vi "DB UI - Config.vi"() -> ()   [LabVIEW 2013]
uses:
  <vilib>/event_ctls.llb/lveventtype.ctl
  Controls/Combo Box.ctl
  <vilib>/Utility/miscctls.llb/LVRowAndColumnTypeDef.ctl
  <vilib>/Utility/miscctls.llb/LVRowAndColumnUnsignedTypeDef.ctl
  Controls/DB - Table Group Enum.ctl
  <vilib>/Utility/miscctls.llb/LVPointTypeDef.ctl
  Controls/DB - OpenClose.ctl
  Controls/DB - Config Table Enum.ctl
  Controls/MCListbox - Enum.ctl
  Controls/Global SRTRS.vi
  Controls/Global CMS.vi
  Controls/Global AMS.vi
  <vilib>/addons/database/Connection.llb/DB Tools Open Connec (String).vi
  <vilib>/addons/database/Connection.llb/Conn Execute.vi
  <vilib>/addons/database/Recordset.llb/Rec Fetch Recordset Data (R).vi
  <vilib>/addons/database/Recordset.llb/Rec Destroy - Connection.vi
  <vilib>/addons/database/_DB Variant To Data/Database Variant To Data.xnode
  <vilib>/addons/database/NI_Database_API.lvlib
panel:
  in  "Application":string
  in  "Records [CaptionOnly]":string caption="Records"
  in  "Header [CaptionOnly]":string caption="Header"
  in  "Tab Control":enum32{"Debug"}(tab)
  out "MHandler":errorcluster
  out "Connection Information":T1={"Connection "="SQL Server 32bit HPEnvy", "Username"="admin", "Password"="admin123"}
  in  "Stop Button":bool
  in  "# of Columns":i32=5
  out "Primary Keys":string[](array[string])=["OrderNo"]
  out "Foreign Keys":string[](array[string])=["OrderNo"]
  out "1st Primary KEY":string
  out "datetime string":string
  out "Changed":bool
  out "SQL Query":string
  out "Extra Event From \"Select Foreign Key\"":bool
  out "IDENTITY COLUMN":string
  out "New Record in UI not in DB":bool
  out "DB.Config.TableGroupType":string="SRTRS.Config.TableGroupType"
  out "Active Cell:Active Cell":T2
  out "# of Columns in DB Table":i32
  out "DB.Config.TableGroup":string="SRTRS.Config.TableGroup"
  in  "CellBG New Cells":u32(colorbox)=16777225
  in  "CellBG Unused Cells":u32(colorbox)=16777238
  in  "CellBG ColHdrs":u32(colorbox)=11776947
  out "Statemachine":errorcluster
  out "Close":errorcluster
  out "Property Node":errorcluster
  out "Foreign Key Selected":string
  out "Type":T3=enum."Value Change"
  out "MCListBox EditCell, Extra Event From  \"Select Foreign Key\"":u32
  out "DB":errorcluster
  in  "Copy":bool
  in  "Database Group":string(combo)
  in  "Save":bool caption="Setup Save"
  in  "Delete":bool caption="Setup Save"
  in  "New":bool caption="Setup Save"
  out "Table Description":string
  in  "Table Name":T4
  in  "Include Inactive":bool
  in  "First Button":bool
  in  "Last Button":bool
  in  "Select Foreign Key":string(combo)="bee"
  in  "Current Record":i32
  in  "Previous Button":bool
  in  "Next Button":bool
  out "Record Count":i32
  in  "Multicolumn Listbox":i32(listbox)=3
  # "Cannot be placed in Tabs, because calling VI only looking at first level."
  # "/"
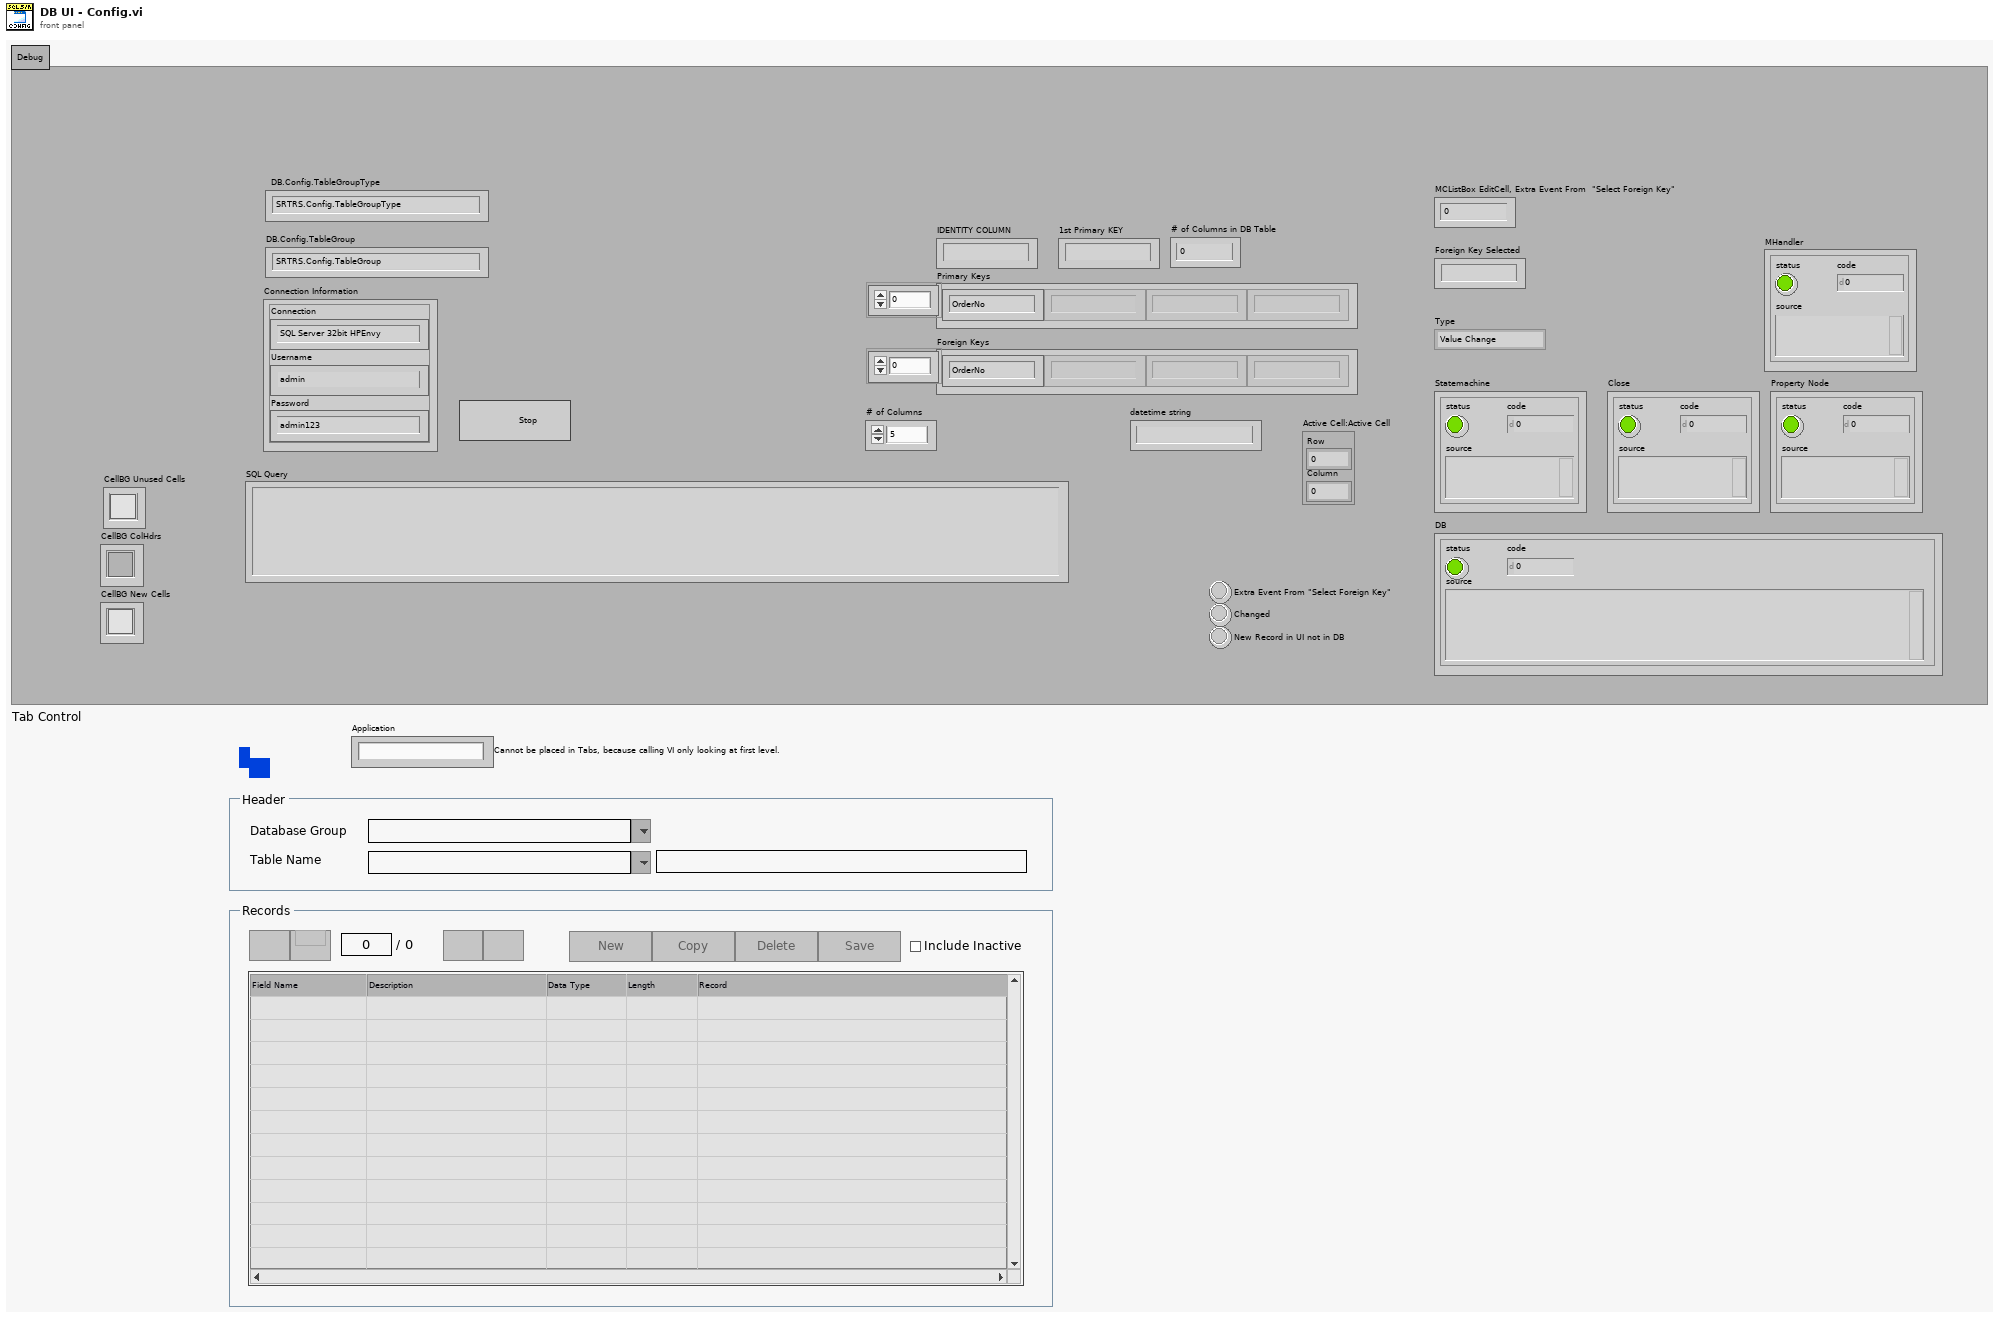
[diagram p1: front panel]
types:
  T1 = cluster{"Connection ":string, "Username":string, "Password":string}
  T2 = typedef "LVRowAndColumnTypeDef.ctl" = cluster{"Row":i32, "Column":i32}
  T3 = typedef "lveventtype.ctl" = enum32{"Null", "Timeout", "Annotation Menu Selection", "Annotation Menu Selection?", "App Instance Close", "App Instance Close?", "Autoscale Range Change", "Bookmark Info Change", "Cell Edit", "Cell Edit?", "Cursor Grab", "Cursor Grab?", "Cursor Menu Selection", "Cursor Menu Selection?", "Cursor Move", "Cursor Release", "Data Change", "Direction Change", "Display State Change", "Drag Ended", "Drag Enter", "Drag Leave", "Drag Over", "Drag Source Update", "Drag Starting", "Drag Starting?", "Drop", "Exec State Change", "Key Down", "Key Down?", "Key Repeat", "Key Repeat?", "Key Up", "Listbox Double Click", "Menu Activation?", "Menu Selection (App)", "Menu Selection? (App)", "Menu Selection (User)", "Mouse Down", "Mouse Down?", "Mouse Enter", "Mouse Leave", "Mouse Move", "Mouse Up", "Mouse Wheel", "NI Security User Change (App)", "Pane Size", "Panel Close", "Panel Close?", "Panel Resize", "Plot Attribute Change", "Scale Range Change", "Shortcut Menu Activation?", "Shortcut Menu Selection (App)", "Shortcut Menu Selection? (App)", "Shortcut Menu Selection (User)", "Tree Double Click", "Tree Drag", "Tree Drag?", "Tree Drop", "Tree Drop?", "Tree Item Close", "Tree Item Close?", "Tree Item Open", "Tree Item Open?", "User Event", "Value Change"}
  T4 = typedef "Combo Box.ctl" = string
  T5 = typedef "DB - OpenClose.ctl" = cluster{"Open":bool, "Close":bool}
  T6 = typedef "LVPointTypeDef.ctl" = cluster{"Horizontal":i16, "Vertical":i16}
  T7 = typedef "DB - Table Group Enum.ctl" = enum16{"SELECT [Description]", "SELECT [TableGroupId]"}
  T8 = typedef "LVRowAndColumnUnsignedTypeDef.ctl" = cluster{"Row":u32, "Column":u32}
  T9 = enum8{"Enabled", "Disabled", "Disabled and Grayed Out"}
  T10 = typedef "Connection Information Cluster.ctl" = cluster{"Connection ":string, "Username":string, "Password":string}
  T11 = typedef "NI_Database_API.lvlib/Conn ObjectReference.ctl" = refnum<k1>
  T12 = typedef "DB - Config Table Enum.ctl" = enum16{"Column Name", "Description", "Type", "Length", "Value (Data)"}
  T13 = typedef "MCListbox - Enum.ctl" = enum16{"Initial (KD?)", "Initial Text", "B4 <Return>", "Now", "Max row count", "Mandatory Fields", "Data Type", "Stored Row, Col, Color"}
  T14 = enum16{"Find FK's Primary Schema.Table", "Find PK's Foreign Schema.Table"}
  T15 = typedef "eventvkey.ctl" = enum16{"ASCII", "Enter", "Return", "Shift", "Ctrl", "Alt", "Cmd", "Opt", "Caps", "NumLock", "Clear", "Break", "Up", "Down", "Left", "Right", "Insert", "Delete", "Home", "End", "PageUp", "PageDown", "Escape", "Help", "Pause", "ScrollLock", "F1", "F2", "F3", "F4", "F5", "F6", "F7", "F8", "F9", "F10", "F11", "F12", "F13", "F14", "F15", "F16", "F17", "F18", "F19", "F20", "F21", "F22", "F23", "F24", "Play", "VolumeUp", "VolumeDown", "Mute", "Two Byte Char"}
  T16 = typedef "LVPoint32TypeDef.ctl" = cluster{"Horizontal":i32, "Vertical":i32}
  T17 = typedef "NI_Database_API.lvlib/Rec ObjectReference.ctl" = refnum<k1>
  T18 = typedef "DB - DB.Schema.Table.ctl" = cluster{"DB":string, "Schema":string, "Table":string}
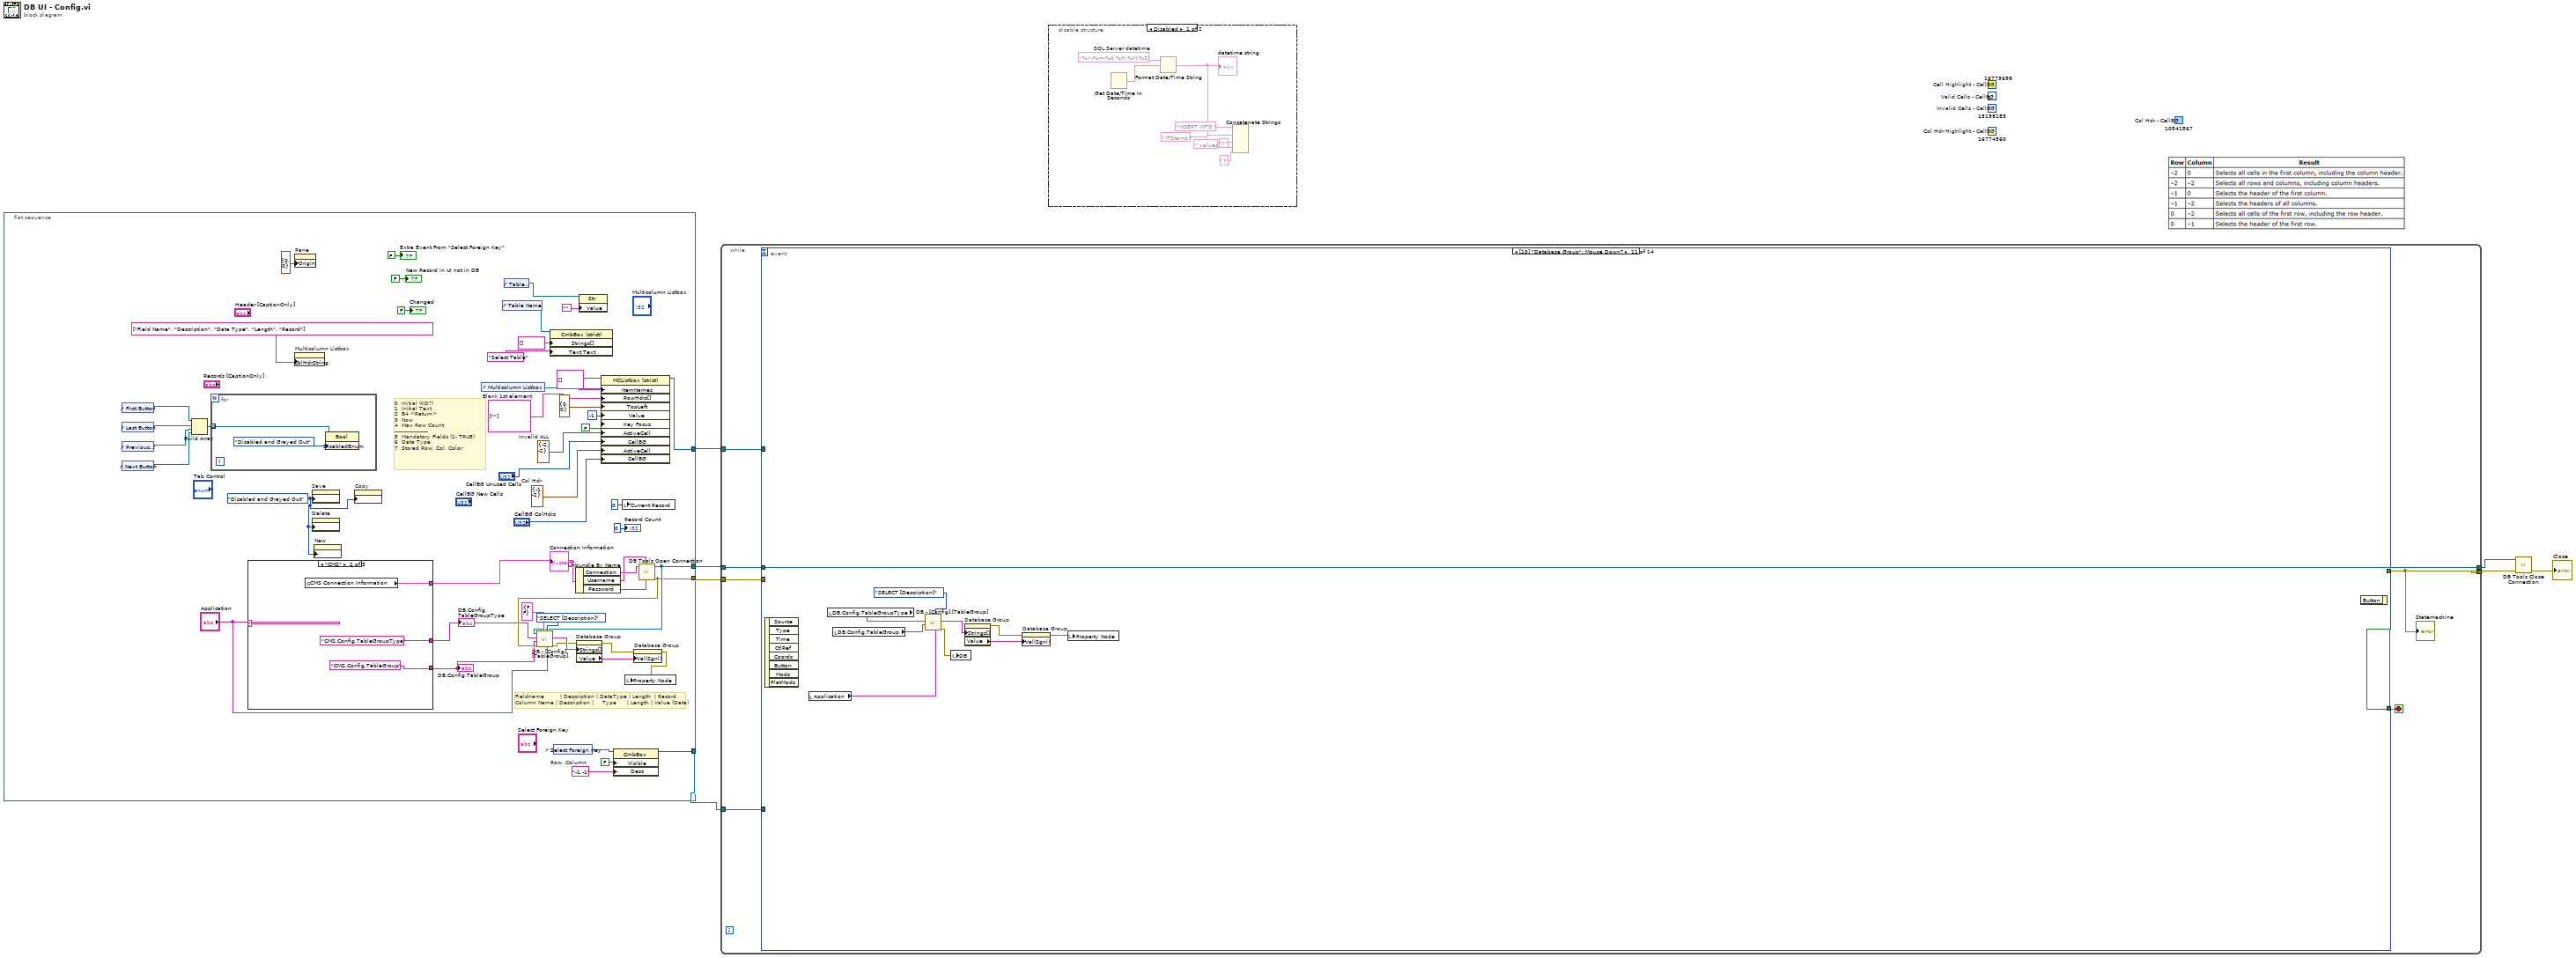
[diagram p0: block diagram]
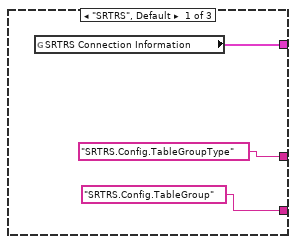
[diagram p3: hidden frame]
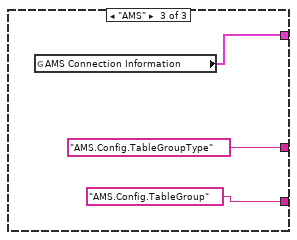
[diagram p4: hidden frame]
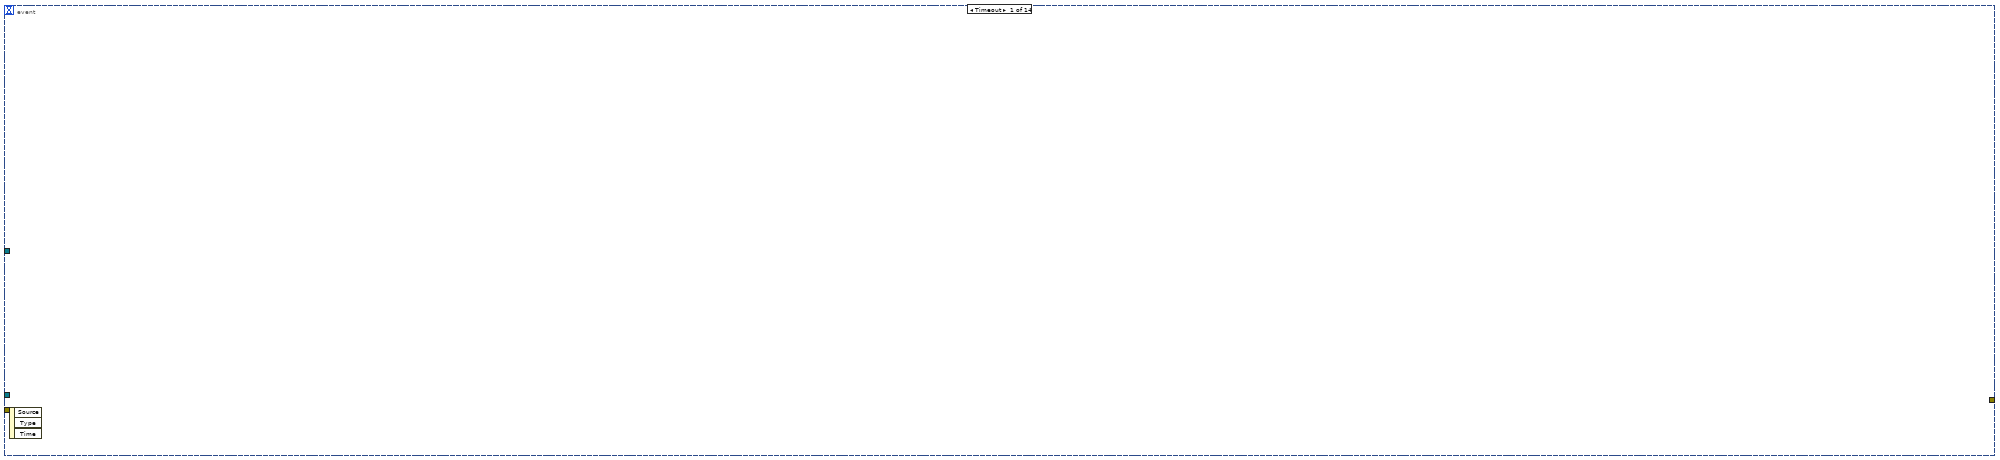
[diagram p5: hidden frame]
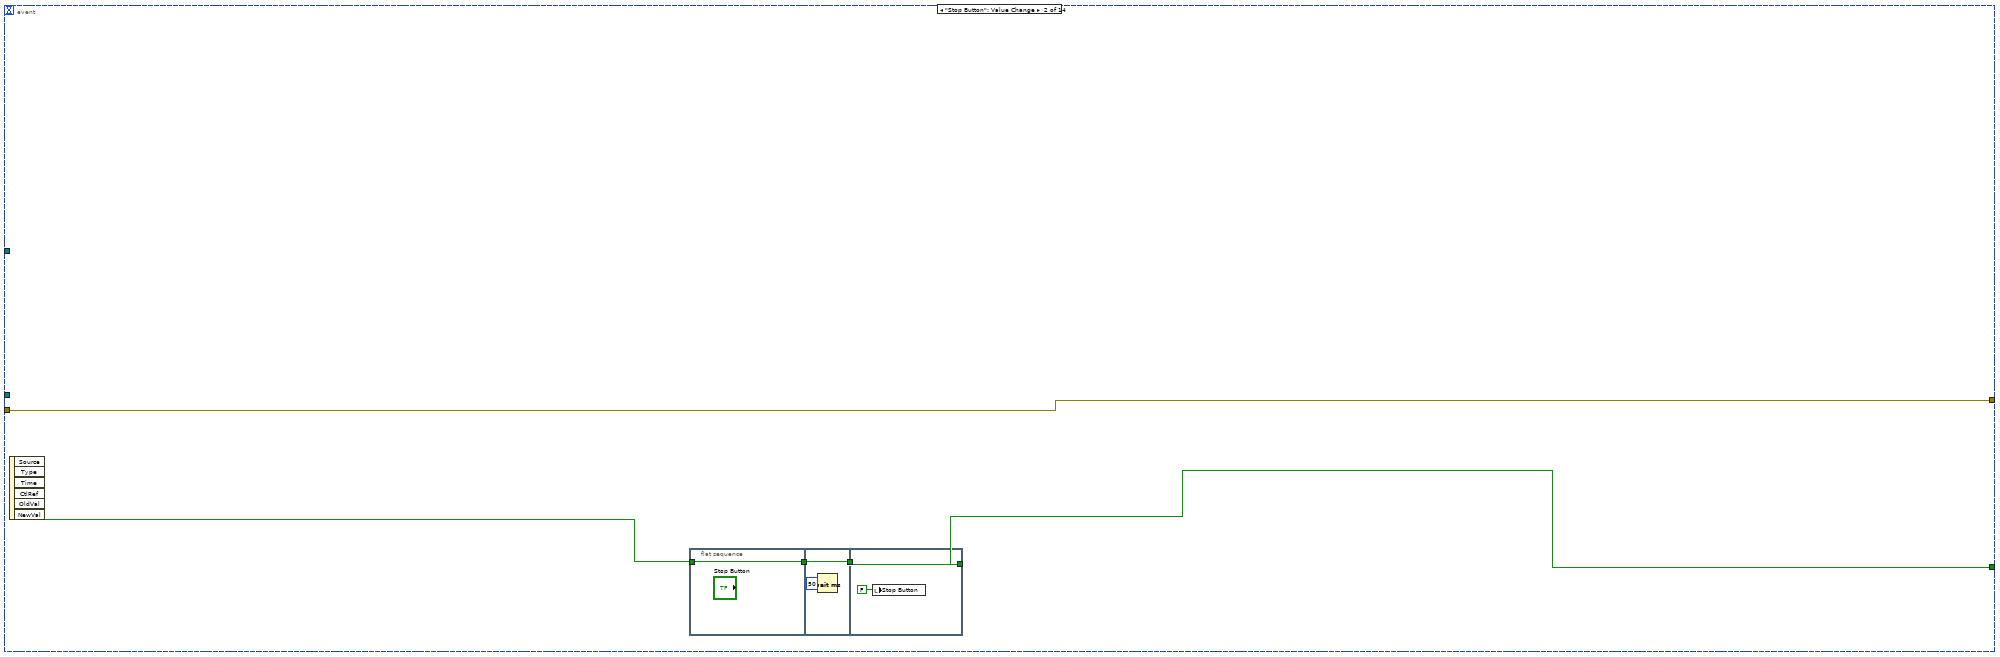
[diagram p6: hidden frame]
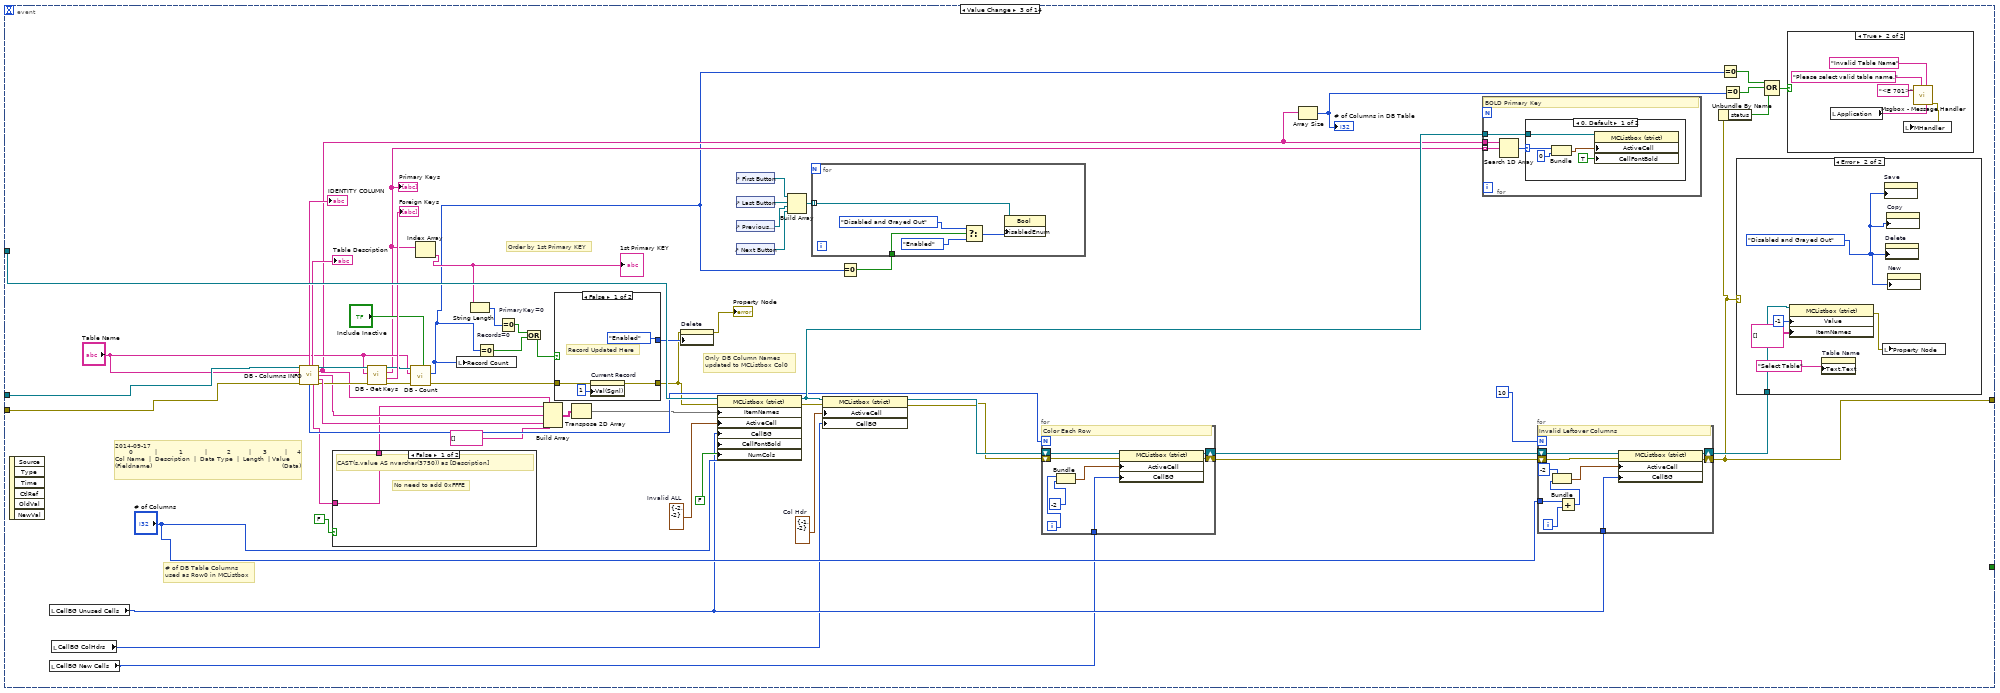
[diagram p7: hidden frame]
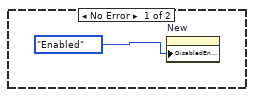
[diagram p9: hidden frame]
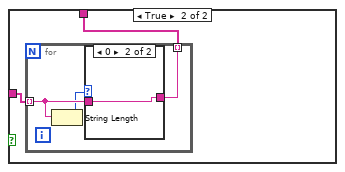
[diagram p10: hidden frame]
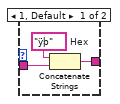
[diagram p11: hidden frame]
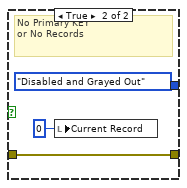
[diagram p12: hidden frame]
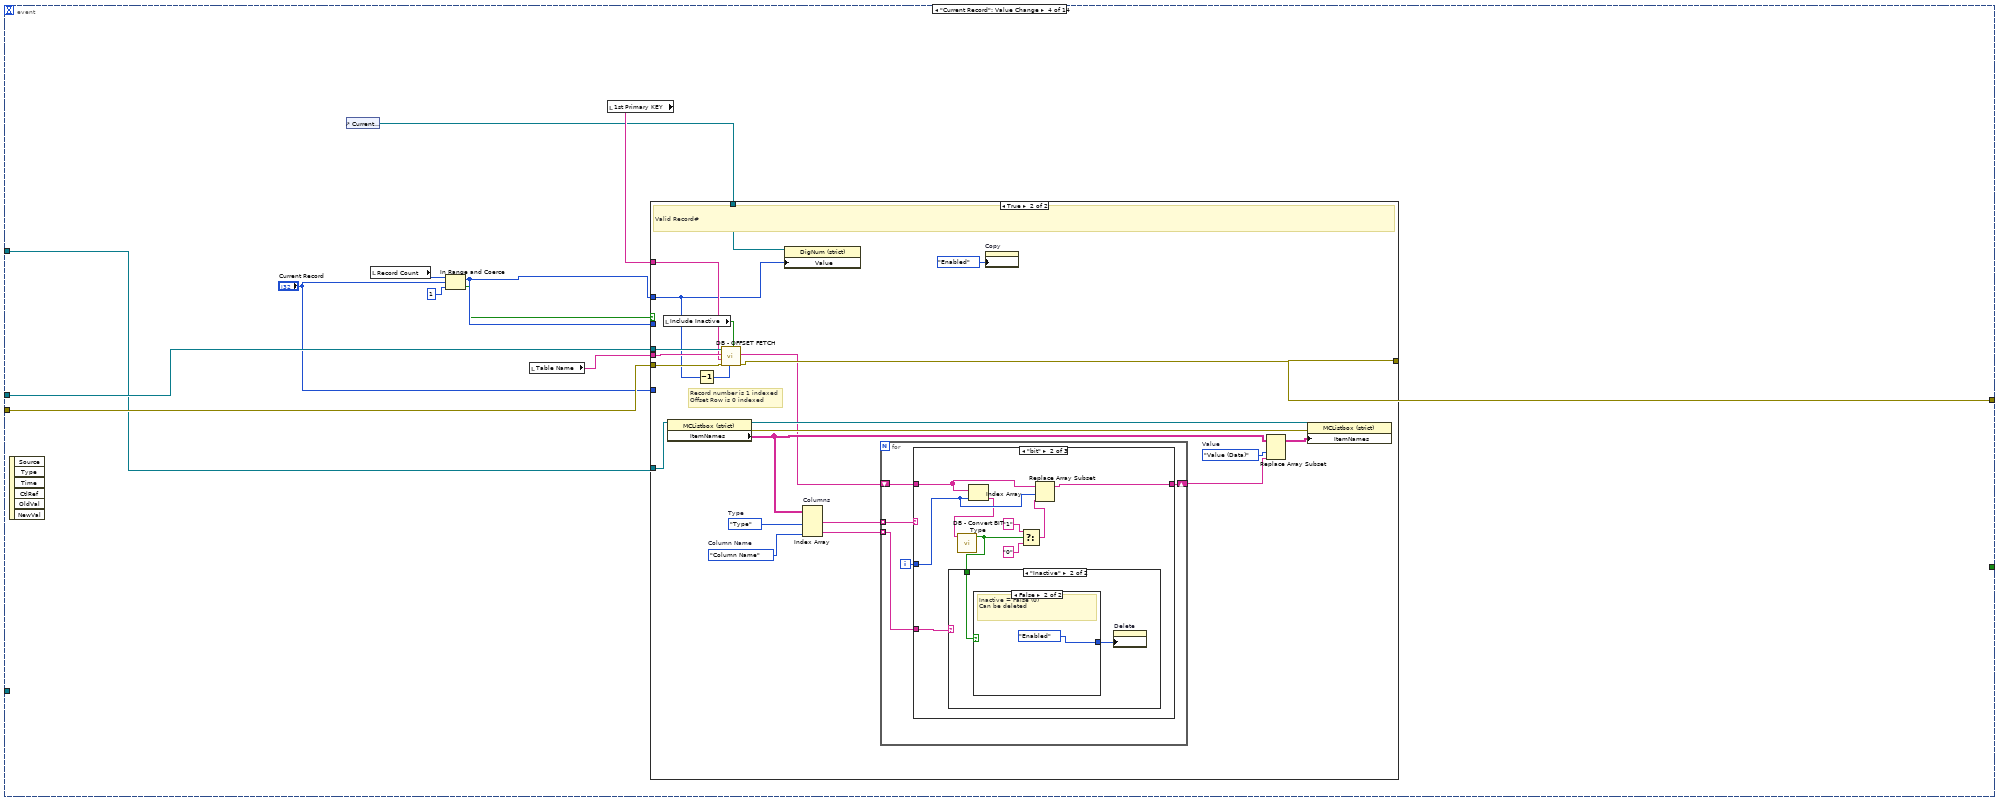
[diagram p14: hidden frame]
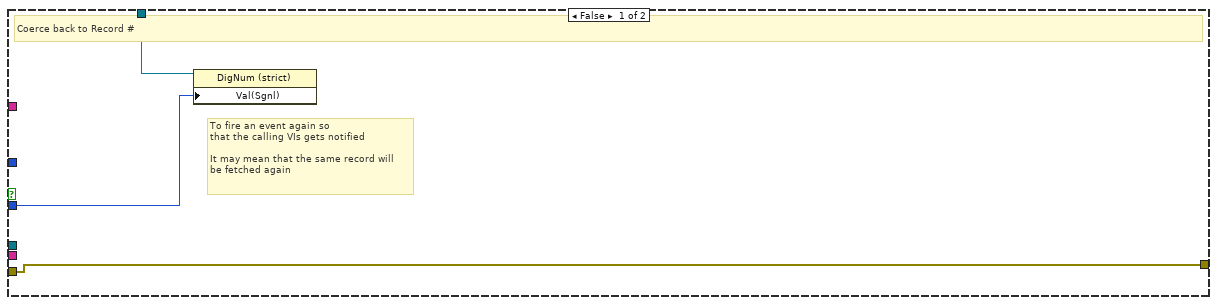
[diagram p15: hidden frame]
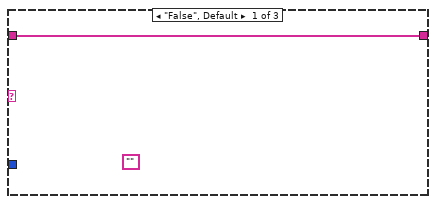
[diagram p16: hidden frame]
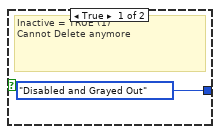
[diagram p18: hidden frame]
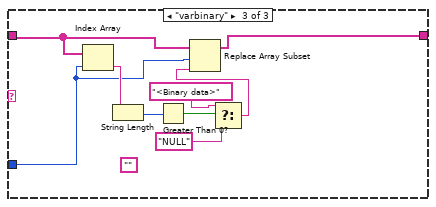
[diagram p19: hidden frame]
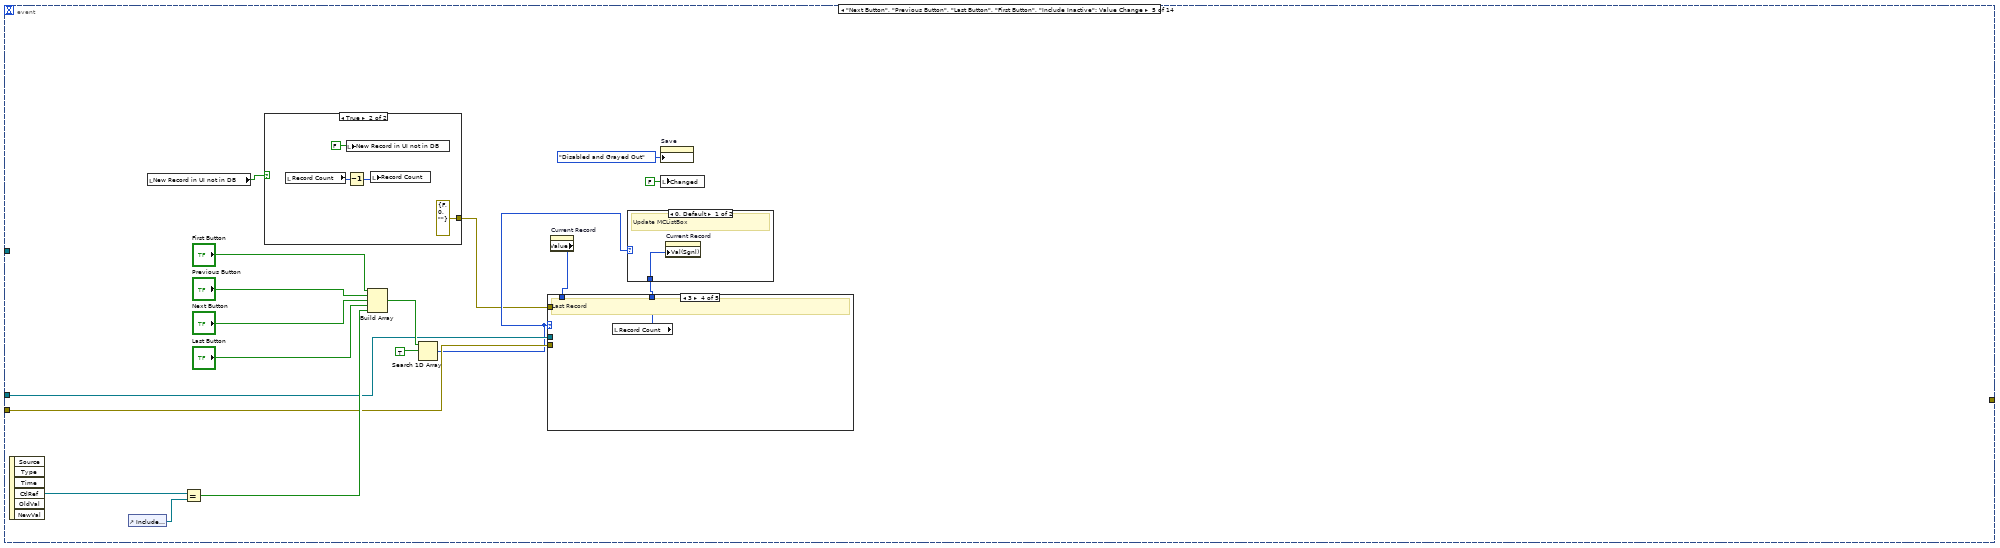
[diagram p20: hidden frame]
diagram:
  (unwired) u32 10541567  # Col Hdr - CellBG
  (unwired) u32 16777226  # Valid Cells - CellBG
  (unwired) u32 15198183  # Invalid Cells - CellBG
  (unwired) u32 16774560  # Col Hdr Highlight - CellBG
  (unwired) u32 16773698  # Cell Highlight - CellBG
  n1 = flat-sequence {
    tunnel: [w18] -> w7
    tunnel: [w52] -> w4
    tunnel: [w17] -> w3
    tunnel: [w49] -> w2
    frame #0 {
      w26 = T2 {"Row"=-1, "Column"=-2}  # Col Hdr
      w27 = T2 {"Row"=-2, "Column"=-2}  # Invalid ALL
      w28 = string[] [""]  # Blank 1st element
      w9 = T9."Disabled and Grayed Out" ("Disabled")
      w47 = "-1,-1"  # Row, Column
      # "Fieldname         | Description | DataType | Length  | Record \nColumn Name | Description |     Type      | Length | Value (Data)"
      # "0  Initial (KD?)\n1  Initial Text\n2  B4 <Return>\n3  Now\n4  Max Row Count\n-------------------\n5  Mandatory Fields (1- TRUE)\n6  Data Type\n7  Stored Row, Col, Color"
      n2 = control-ref of="First Button"() -> (w43:refnum<vi>)
      n3 = control-ref of="Last Button"() -> (w42:refnum<vi>)
      n4 = control-ref of="Previous Button"() -> (w41:refnum<vi>)
      n5 = control-ref of="Next Button"() -> (w40:refnum<vi>)
      n6 = Build Array(w43, w42, w41, w40) -> (w44:refnum<vi>[])
      n7 = for {
        tunnel: w44 -> [w67] mode=indexing
        n8 = property class="Bool"(reference=w67, "DisabledEnum"=T9."Disabled and Grayed Out" ("Disabled")) -> ()  [unwired: 1 in, 2 out]
      }
      n9 = case shown="\"CMS\"" "Application" {
        tunnel: [w59 w62 w63] -> w21
        tunnel: ["SRTRS.Config.TableGroupType" ("DB.Schema.Table\nDB.Config.TableGroupType") "CMS.Config.TableGroupType" ("DB.Schema.Table\nDB.Config.TableGroupType") "AMS.Config.TableGroupType" ("DB.Schema.Table\nDB.Config.TableGroupType")] -> w20
        tunnel: ["SRTRS.Config.TableGroup" ("DB.Schema.Table\nDB.Config.TableGroup") "CMS.Config.TableGroup" ("DB.Schema.Table\nDB.Config.TableGroup") "AMS.Config.TableGroup" ("DB.Schema.Table\nDB.Config.TableGroup")] -> w10
        frame "SRTRS", Default {
          n10 = global read "Global SRTRS.vi" "SRTRS Connection Information"() -> (w59:T10)
        }
        frame "CMS" {
          n11 = global read "Global CMS.vi" "CMS Connection Information"() -> (w62:T10)
        }
        frame "AMS" {
          n12 = global read "Global AMS.vi" "AMS Connection Information"() -> (w63:T10)
        }
      }
      "Connection Information" <- w21
      "DB.Config.TableGroupType" <- w20
      "DB.Config.TableGroup" <- w10
      n13 = property on="Pane" class="Pane"("Origin"=T6 {"Horizontal"=0, "Vertical"=0}) -> ()  [unwired: 2 in, 2 out]
      n14 = property on="Multicolumn Listbox" class="MCListbox (strict)"("ColHdrString"=string[] ["Field Name", "Description", "Data Type", "Length", "Record"] ("Column Header Strings[]")) -> ()  [unwired: 2 in, 2 out]
      n15 = property on="Save" class="Bool"("DisabledEnum"=w9) -> ()  [unwired: 2 in, 2 out]
      n16 = property on="Delete" class="Bool"("DisabledEnum"=w9) -> ()  [unwired: 2 in, 2 out]
      n17 = property on="New" class="Bool"("DisabledEnum"=w9) -> ()  [unwired: 2 in, 2 out]
      n18 = property on="Copy" class="Bool"("DisabledEnum"=w9) -> ()  [unwired: 2 in, 2 out]
      n19 = control-ref of="Multicolumn Listbox"() -> (w22:refnum<vi>)
      n20 = control-ref of="Table Name"() -> (w39:refnum<vi>)
      n21 = control-ref of="Table Description"() -> (w37:refnum<vi>)
      n22 = property on="Property Node" class="CmbBox (strict)"(reference=w39, "Strings[]"=string[] [] ("Strings []"), "Text.Text"="Select Table") -> ()  [unwired: 1 in, 2 out]
      n23 = control-ref of="Select Foreign Key"() -> (w50:refnum<vi>)
      n24 = Unbundle By Name(w21) -> ("Connection"=w55:string, "Username"=w54:string, "Password"=w53:string)
      n25 = property on="Property Node" class="Str"(reference=w37, "Value"="") -> ()  [unwired: 1 in, 2 out]
      n26 = property on="Property Node" class="MCListbox (strict)"(reference=w22, "ItemNames"=string[][] [] ("Item Names"), "RowHdrs[]"=w28, "TopLeft"=T8 {"Row"=0, "Column"=0} ("Top Left Visible Cell"), "Value"=-1, "Key Focus"=FALSE, "ActiveCell"=w27, "CellBG"="CellBG Unused Cells", "ActiveCell"=w26, "CellBG"="CellBG ColHdrs") -> (reference out=w52:refnum<vi>)  [unwired: 1 in, 1 out]
      n27 = property class="CmbBox"(reference=w50, "Visible"=FALSE, "Desc"=w47) -> (reference out=w49:refnum<vi>)  [unwired: 1 in, 1 out]
      n28 = local write "Current Record"(0 ("Current Record")) -> ()
      n29 = call-poly <vilib>:"DB Tools Open Connection.vi"("password"=w53, "userID"=w54, "connection information"=w55) -> ("error out"=w17:errorcluster, "connection reference"=w18:T11)  [unwired: 5 in]
      n30 = call "DB - [Config].[TableGroup].vi"("Application"="Application", "Table Group Enum"=DB_-_Table_Group_Enum."SELECT [Description]", "DB Connection"=T5 {"Open"=FALSE, "Close"=FALSE}, "error in (no error)"=w17, "DB.Config.TableGroup"=w10, "DB.Config.TableGroupType"=w20, "connection reference"=w18) -> ("SUMMARY"=w16:errorcluster, "data"=w31:string[])  [unwired: 2 in, 1 out]
      n31 = property on="Database Group" class="CmbBox"(error in=w16, "Strings[]"=w31) -> (error out=w25:errorcluster, "Value"=w24:string)  [unwired: 1 in, 1 out]
      n32 = property on="Database Group" class="CmbBox"(error in=w25, "Val(Sgnl)"=w24) -> (error out=w15:errorcluster)  [unwired: 1 in, 1 out]
      n33 = local write "Property Node"(w15) -> ()
      "Extra Event From \"Select Foreign Key\"" <- FALSE ("Extra Event From \"Select Foreign Key Value Changed\"")
      "Record Count" <- 0 ("Record Count")
      "New Record in UI not in DB" <- FALSE ("New Record in UI not in DB")
      "Changed" <- FALSE ("Changed")
    }
  }
  n34 = while {
    tunnel: w7 -> [w69]
    tunnel: [w69] -> w6
    tunnel: [w68] -> w5
    tunnel: w3 -> [w72]
    tunnel: w4 -> [w71]
    tunnel: w2 -> [w70]
    stop <- w73 stop-if-true
    n35 = event shown="[10] \"Database Group\": Mouse Down?" {
      selector: _ -> [_ _ _ _ _ _ _ _ _ _ _ _ _ _]
      dyn-events: _ -> [_ _ _ _ _ _ _ _ _ _ _ _ _ _]
      timeout: _ -> [_ _ _ _ _ _ _ _ _ _ _ _ _ _]
      tunnel: [_ w76 _ _ _ _ _ _ _ _ _ _ _ _] -> w73
      tunnel: w69 -> [_ _ w129 w216 w275 _ w367 _ _ w619 _ _ _ w806]
      tunnel: [_ w78 w90 w213 _ _ _ _ _ w581 _ _ _ _] -> w68
      tunnel: w72 -> [_ w78 w126 w215 w274 _ w366 _ _ _ _ _ _ _]
      tunnel: w71 -> [_ _ w138 w212 _ w308 _ _ w535 _ _ w727 w779 _]
      tunnel: w70 -> [_ _ _ _ _ _ w376 _ _ _ _ _ w781 _]
      event Timeout {
        n36 = event-data() -> ()  [unwired: 1 in, 3 out]
      }
      event "Stop Button": Value Change {
        n37 = event-data() -> ("NewVal"=w77:bool)  [unwired: 1 in, 5 out]
        n38 = flat-sequence {
          tunnel: w77 -> [w79]
          tunnel: [w79] -> w74
          tunnel: [w80] -> w75
          tunnel: w74 -> [w80]
          tunnel: [w82] -> w76
          tunnel: w75 -> [w82]
          frame #0 {
          }
          frame #1 {
            n39 = Wait (ms)(milliseconds to wait=u32 50) -> ()  [unwired: 1 out]
          }
          frame #2 {
            n40 = local write "Stop Button"(FALSE ("Stop Button")) -> ()
          }
        }
      }
      event Value Change {
        w130 = T2 {"Row"=-1, "Column"=-2}  # Col Hdr
        w143 = T2 {"Row"=-2, "Column"=-2}  # Invalid ALL
        # "2014-09-17\n       0           |           1           |          2         |      3         |     4\nCol Name  |  Description  |  Data Type  |  Length  | Value \n(Fieldname)                                                                 (Data)"
        # "Only DB Column Names \nupdated to MCListbox Col0"
        # "Order by 1st Primary KEY"
        # "# of DB Table Columns\nused as Row0 in MCListbox"
        n41 = event-data() -> ()  [unwired: 1 in, 6 out]
        n42 = local read "CellBG Unused Cells"() -> (w93:u32)
        n43 = local read "CellBG New Cells"() -> (w91:u32)
        n44 = local read "CellBG ColHdrs"() -> (w92:u32)
        n45 = call "DB - Columns INFO.vi"("Refnum in"=w129, "DB.dbo.Table"="Table Name", "error in (no error)"=w126) -> ("IDENTITY COLUMN"=→"IDENTITY COLUMN":string, "Table Description"=→"Table Description":string, "Refnum out"=w128:T11, "COLUMN_NAME"=w94:string[], "DATA_TYPE"=w121:string[], "PRECISION"=w127:string[], "COUNT"=w108:i32, "MS_Description"=w107:string[], "error out"=w125:errorcluster)  [unwired: 4 in]
        n46 = case shown="False" FALSE {
          tunnel: [w156 w158] -> w98
          tunnel: w107 -> [w156 w157]
          frame False {
            # "No need to add 0xFFFE"
            # "CAST(s.value AS nvarchar(3750)) as [Description]"
          }
          frame True {
            n47 = for {
              tunnel: w157 -> [w160] mode=indexing
              tunnel: [w161] -> w158 mode=indexing
              n48 = String Length(string=w160) -> (length=w159:i32)
              n49 = case shown="0" w159 {
                tunnel: [w163 w165] -> w161
                tunnel: w160 -> [w162 w165]
                frame 1, Default {
                  w164 = "ÿþ"  # Hex
                  n50 = Concatenate Strings(w164, w162) -> (w163:string)
                }
                frame 0 {
                }
              }
            }
          }
        }
        n51 = call "DB - Get Keys.vi"("error in (no error)"=w125, "DB.Schema.Table"="Table Name", "Refnum in"=w128) -> ("error out"=w135:errorcluster, "Foreign Keys"=→"Foreign Keys":string[], "Primary Key"=w95:string[], "Refnum out"=w136:T11)  [unwired: 5 in]
        "Primary Keys" <- w95
        n52 = call "DB - Count.vi"("Include Inactive"="Include Inactive", "error in (no error)"=w135, "DB.dbo.Table"="Table Name", "Refnum in"=w136) -> ("error out"=w122:errorcluster, "COUNT"=w88:i32)  [unwired: 5 in, 1 out]
        n53 = Index Array(array=w95) -> (element=w114:string)  [unwired: 1 in]
        "1st Primary KEY" <- w114
        n54 = local write "Record Count"(w88) -> ()
        n55 = String Length(string=w114) -> (length=w113:i32)
        n56 = Equal To 0? "Records=0"(x=w88) -> (x = 0?=w111:bool)
        n57 = Equal To 0? "PrimaryKey=0"(x=w113) -> (x = 0?=w112:bool)
        n58 = Or(x=w112, y=w111) -> (x .or. y?=w110:bool)
        n59 = Build Array(w94, w98, w121, w127, string[] [] ("element")) -> (w109:string[][])
        n60 = case shown="False" w110 {
          tunnel: w122 -> [w173 w177]
          tunnel: [w172 w177] -> w101
          tunnel: [T9."Enabled" ("Disabled") T9."Disabled and Grayed Out" ("Disabled")] -> w103
          frame False {
            # "Record Updated Here"
            n61 = property on="Current Record" class="DigNum (strict)"(error in=w173, "Val(Sgnl)"=1) -> (error out=w172:errorcluster)  [unwired: 1 in, 1 out]
          }
          frame True {
            # "No Primary KEY\nor No Records"
            n62 = local write "Current Record"(0 ("Current Record")) -> ()
          }
        }
        n63 = Transpose 2D Array(2D array=w109) -> (transposed array=w96:string[][])
        n64 = property on="Delete" class="Bool"(error in=w101, "DisabledEnum"=w103) -> (error out=→"Property Node":errorcluster)  [unwired: 1 in, 1 out]
        n65 = property on="Property Node" class="MCListbox (strict)"(reference=w138, error in=w101, "ItemNames"=w96, "ActiveCell"=w143, "CellBG"=w93, "CellFontBold"=FALSE ("Active Cell:Cell Font:Bold"), "NumCols"="# of Columns") -> (reference out=w134:refnum<vi>, error out=w132:errorcluster)
        n66 = control-ref of="First Button"() -> (w120:refnum<vi>)
        n67 = control-ref of="Last Button"() -> (w119:refnum<vi>)
        n68 = control-ref of="Previous Button"() -> (w118:refnum<vi>)
        n69 = control-ref of="Next Button"() -> (w117:refnum<vi>)
        n70 = Build Array(w120, w119, w118, w117) -> (w116:refnum<vi>[])
        n71 = property on="Property Node" class="MCListbox (strict)"(reference=w134, error in=w132, "ActiveCell"=w130, "CellBG"=w92) -> (reference out=w133:refnum<vi>, error out=w131:errorcluster)
        n72 = Equal To 0?(x=w88) -> (x = 0?=w115:bool)
        n73 = for {
          tunnel: w116 -> [w170] mode=indexing
          tunnel: w115 -> [w169]
          n74 = Select(t=T9."Disabled and Grayed Out" ("Disabled"), s=w169, f=T9."Enabled" ("Disabled")) -> (s? t:f=w166:T9)
          n75 = property class="Bool"(reference=w170, "DisabledEnum"=w166) -> ()  [unwired: 1 in, 2 out]
        }
        n76 = for {
          N: w108 -> [_]
          tunnel: w91 -> [w199]
          shift-right: [w203] -> w142
          shift-left: w131 -> [w204]
          shift-right: [w197] -> w140
          shift-left: w133 -> [w198]
          i -> [w202]
          # "Color Each Row"
          n77 = Bundle(w202, -2) -> (w200:cluster{i32, i32})  [unwired: 1 in]
          n78 = property on="Property Node" class="MCListbox (strict)"(reference=w198, error in=w204, "ActiveCell"=w200, "CellBG"=w199) -> (reference out=w197:refnum<vi>, error out=w203:errorcluster)
        }
        n79 = Array Size(array=w94) -> (size(s)=w89:i32)
        "# of Columns in DB Table" <- w89
        n80 = for {
          tunnel: w95 -> [w181] mode=indexing
          tunnel: w94 -> [w180]
          tunnel: w134 -> [w178]
          # "BOLD Primary Key"
          n81 = Search 1D Array(1D array=w180, element=w181) -> (index of element=w179:i32)  [unwired: 1 in]
          n82 = case shown="0, Default" w179 {
            selector: w179 -> [w185 _]
            tunnel: w178 -> [w186 _]
            frame 0, Default {
              n83 = Bundle("index of element"=w185, 0) -> (w183:cluster{"index of element":i32, i32})  [unwired: 1 in]
              n84 = property on="Property Node" class="MCListbox (strict)"(reference=w186, "ActiveCell"=w183, "CellFontBold"=TRUE ("Active Cell:Cell Font:Bold")) -> ()  [unwired: 1 in, 2 out]
            }
            frame -1 {
            }
          }
        }
        n85 = for {
          N: 10 -> [_]
          tunnel: w93 -> [w192]
          tunnel: "# of Columns" -> [w190]
          shift-right: [w195] -> w90
          shift-left: w142 -> [w196]
          shift-right: [w187] -> w99
          shift-left: w140 -> [w188]
          i -> [w191]
          # "Invalid Leftover Columns"
          n86 = Add(x=w190, y=w191) -> (x+y=w189:i32)
          n87 = Bundle(-2, w189) -> (w194:cluster{i32, i32})  [unwired: 1 in]
          n88 = property on="Property Node" class="MCListbox (strict)"(reference=w188, error in=w196, "ActiveCell"=w194, "CellBG"=w192) -> (reference out=w187:refnum<vi>, error out=w195:errorcluster)
        }
        n89 = Unbundle By Name(w90) -> ("status"=w85:bool)
        n90 = Equal To 0?(x=w88) -> (x = 0?=w87:bool)
        n91 = Equal To 0?(x=w89) -> (x = 0?=w86:bool)
        n92 = case shown="Error" w90 {
          tunnel: w99 -> [_ w155]
          frame No Error {
            n93 = property on="New" class="Bool"("DisabledEnum"=T9."Enabled" ("Disabled")) -> ()  [unwired: 2 in, 2 out]
          }
          frame Error {
            w150 = T9."Disabled and Grayed Out" ("Disabled")
            n94 = property on="Property Node" class="MCListbox (strict)"(reference=w155, "Value"=-1, "ItemNames"=string[][] [] ("Item Names")) -> (error out=w152:errorcluster)  [unwired: 1 in, 1 out]
            n95 = property on="Table Name" class="CmbBox (strict)"("Text.Text"="Select Table") -> ()  [unwired: 2 in, 2 out]
            n96 = local write "Property Node"(w152) -> ()
            n97 = property on="Save" class="Bool"("DisabledEnum"=w150) -> ()  [unwired: 2 in, 2 out]
            n98 = property on="Delete" class="Bool"("DisabledEnum"=w150) -> ()  [unwired: 2 in, 2 out]
            n99 = property on="Copy" class="Bool"("DisabledEnum"=w150) -> ()  [unwired: 2 in, 2 out]
            n100 = property on="New" class="Bool"("DisabledEnum"=w150) -> ()  [unwired: 2 in, 2 out]
          }
        }
        n101 = Compound Arithmetic op=OR(w87, w86, w85) -> (w84:bool)
        n102 = case shown="True" w84 {
          frame False {
          }
          frame True {
            n103 = local read "Application"() -> (w144:string)
            n104 = call "Msgbox - Message Handler.vi"("Application (Default SRTRS)"=w144, "Short Description (When DB Not Available)"="Invalid Table Name", "Description (When DB Not Available)"="Please select valid table name.", "<.?....> Message Code"="<E 701>") -> ("MHandler Error"=w145:errorcluster)  [unwired: 5 in, 2 out]
            n105 = local write "MHandler"(w145) -> ()
          }
        }
      }
      event "Current Record": Value Change {
        n106 = event-data() -> ()  [unwired: 1 in, 6 out]
        n107 = control-ref of="Current Record"() -> (w207:refnum<vi>)
        n108 = local read "Record Count"() -> (w208:i32)
        n109 = In Range and Coerce(upper limit=w208, x="Current Record", lower limit=1) -> (coerced(x)=w209:i32, In Range?=w205:bool)
        n110 = local read "Table Name"() -> (w211:T4)
        n111 = local read "1st Primary KEY"() -> (w214:string)
        n112 = case shown="True" w205 {
          tunnel: w216 -> [_ w241]
          tunnel: w215 -> [w219 w240]
          tunnel: w211 -> [_ w239]
          tunnel: w214 -> [_ w238]
          tunnel: w209 -> [_ w231]
          tunnel: [w219 w237] -> w213
          tunnel: w212 -> [_ w236]
          tunnel: "Current Record" -> [_ _]
          tunnel: w209 -> [w217 _]
          tunnel: w207 -> [w218 w232]
          frame False {
            # "To fire an event again so\nthat the calling VIs gets notified\n\nIt may mean that the same record will \nbe fetched again"
            # "Coerce back to Record #"
            n113 = property class="DigNum (strict)"(reference=w218, "Val(Sgnl)"=w217) -> ()  [unwired: 1 in, 2 out]
          }
          frame True {
            w222 = DB_-_Config_Table_Enum."Column Name"  # Column Name
            w226 = DB_-_Config_Table_Enum."Value (Data)"  # Value
            w229 = DB_-_Config_Table_Enum."Type"  # Type
            # "Record number is 1 indexed\nOffset Row is 0 indexed"
            # "Valid Record#"
            n114 = local read "Include Inactive"() -> (w230:bool)
            n115 = property class="MCListbox (strict)"(reference=w236) -> (reference out=w235:refnum<vi>, error out=w234:errorcluster, "ItemNames"=w227:string[][])  [unwired: 1 in]
            n116 = Decrement(x=w231) -> (x-1=w233:i32)
            n117 = call "DB - OFFSET FETCH.vi"("Include Inactive"=w230, "OFFSET ROW"=w233, "error in (no error)"=w240, "Column to Order BY"=w238, "DB.dbo.Table"=w239, "Refnum in"=w241) -> ("error out"=w237:errorcluster, "Data"=w225:string[])  [unwired: 3 in, 1 out]
            n118 = property class="DigNum (strict)"(reference=w232, "Value"=w231) -> ()  [unwired: 1 in, 2 out]
            n119 = Index Array "Columns"(array=w227, index (col) #1=w229, index (col) #2=w222) -> (element #1=w228:string[], element #2=w221:string[])  [unwired: 2 in]
            n120 = for {
              tunnel: w228 -> [w246] mode=indexing
              shift-right: [w244] -> w224
              shift-left: w225 -> [w245]
              tunnel: w221 -> [w242] mode=indexing
              i -> [w243]
              n121 = case shown="\"bit\"" w246 {
                tunnel: w245 -> [w247 w256 w268]
                tunnel: [w247 w254 w269] -> w244
                tunnel: w243 -> [_ w255 w262]
                tunnel: w242 -> [_ w248 _]
                frame "False", Default {
                  (unwired) ""
                }
                frame "bit" {
                  n122 = Index Array(array=w256, index=w255) -> (element=w253:string)
                  n123 = call "DB - Convert BIT Type.vi"("BIT Type (eg Inactive)"=w253) -> ("Boolean"=w249:bool)  [unwired: 2 in, 2 out]
                  n124 = case shown="\"Inactive\"" w248 {
                    tunnel: w249 -> [_ w258]
                    frame "False", Default {
                    }
                    frame "Inactive" {
                      n125 = case shown="False" w258 {
                        tunnel: [T9."Disabled and Grayed Out" ("Disabled") T9."Enabled" ("Disabled")] -> w257
                        frame True {
                          # "Inactive = TRUE (1)\nCannot Delete anymore"
                        }
                        frame False {
                          # "Inactive = False (0)\nCan be deleted"
                        }
                      }
                      n126 = property on="Delete" class="Bool"("DisabledEnum"=w257) -> ()  [unwired: 2 in, 2 out]
                    }
                  }
                  n127 = Select(t="1", s=w249, f="0") -> (s? t:f=w250:string)
                  n128 = Replace Array Subset(array=w256, new element=w250, index=w255) -> (w254:string[])
                }
                frame "varbinary" {
                  (unwired) ""
                  n129 = Index Array(array=w268, index=w262) -> (element=w267:string)
                  n130 = String Length(string=w267) -> (length=w266:i32)
                  n131 = Greater Than 0?(x=w266) -> (x > 0?=w265:bool)
                  n132 = Select(t="<Binary data>", s=w265, f="NULL") -> (s? t:f=w263:string)
                  n133 = Replace Array Subset(array=w268, new element=w263, index=w262) -> (w269:string[])
                }
              }
            }
            n134 = property on="Copy" class="Bool"("DisabledEnum"=T9."Enabled" ("Disabled")) -> ()  [unwired: 2 in, 2 out]
            n135 = Replace Array Subset(array=w227, new element=w224, index (col)=w226) -> (w223:string[][])  [unwired: 1 in]
            n136 = property class="MCListbox (strict)"(reference=w235, error in=w234, "ItemNames"=w223) -> ()  [unwired: 2 out]
          }
        }
      }
      event "Next Button", "Previous Button", "Last Button", "First Button", "Include Inactive": Value Change {
        n137 = event-data() -> ("CtlRef"=w278:refnum<vi>)  [unwired: 1 in, 5 out]
        n138 = control-ref of="Include Inactive"() -> (w277:refnum<vi>)
        n139 = local read "New Record in UI not in DB"() -> (w272:bool)
        n140 = Equal?(x=w278, y=w277) -> (x = y?=w276:bool)
        n141 = case shown="True" w272 {
          tunnel: [_ errorcluster {"status"=FALSE, "code"=0, "source"=""} ("error constant")] -> w271
          frame False {
          }
          frame True {
            n142 = local read "Record Count"() -> (w290:i32)
            n143 = local write "New Record in UI not in DB"(FALSE ("New Record in UI not in DB")) -> ()
            n144 = Decrement(x=w290) -> (x-1=w289:i32)
            n145 = local write "Record Count"(w289) -> ()
          }
        }
        n146 = Build Array("First Button", "Previous Button", "Next Button", "Last Button", w276) -> (w283:bool[])
        n147 = Search 1D Array(1D array=w283, element=TRUE) -> (index of element=w273:i32)  [unwired: 1 in]
        n148 = property on="Current Record" class="DigNum (strict)"() -> ("Value"=w287:i32)  [unwired: 2 in, 2 out]
        n149 = case shown="3" w273 {
          tunnel: w287 -> [_ w295 w297 _ w302]
          tunnel: [1 w294 w296 w298 w302] -> w286
          tunnel: w275 -> [_ _ _ _ _]
          tunnel: w274 -> [_ _ _ _ _]
          tunnel: w271 -> [_ _ _ _ _]
          frame 0, Default {
            # "1st Record"
          }
          frame 1 {
            # "Previous"
            n150 = Decrement(x=w295) -> (x-1=w294:i32)
          }
          frame 2 {
            # "Next"
            n151 = Increment(x=w297) -> (x+1=w296:i32)
          }
          frame 3 {
            # "Last Record"
            n152 = local read "Record Count"() -> (w298:i32)
          }
          frame 4 {
            # "Refresh the entireTable because we need to update # of Records also"
            # "Include Invalid"
            n153 = control-ref of="Table Name"() -> (w300:refnum<vi>)
            n154 = property on="Property Node" class="CmbBox (strict)"(reference=w300) -> (reference out=w299:refnum<vi>, "Value"=w301:T4)  [unwired: 1 in, 1 out]
            n155 = property on="Property Node" class="CmbBox (strict)"(reference=w299, "Val(Sgnl)"=w301) -> ()  [unwired: 1 in, 2 out]
          }
        }
        n156 = case shown="0, Default" w273 {
          tunnel: w286 -> [w292 _]
          frame 0, Default {
            # "Update MCListBox"
            n157 = property on="Current Record" class="DigNum (strict)"("Val(Sgnl)"=w292) -> ()  [unwired: 2 in, 2 out]
          }
          frame 4 {
            # "Event already FIRED in Select Table"
          }
        }
        n158 = local write "Changed"(FALSE ("Changed")) -> ()
        n159 = property on="Save" class="Bool"("DisabledEnum"=T9."Disabled and Grayed Out" ("Disabled")) -> ()  [unwired: 2 in, 2 out]
      }
      event "Multicolumn Listbox": Key Down {
        # "Move EditPos to next available Cell on Return, Enter, TAB"
        n160 = event-data() -> ("Char"=w306:i16, "VKey"=w307:T15)  [unwired: 1 in, 8 out]
        n161 = case shown="\"Enter\", \"Return\"" w307 {
          tunnel: [FALSE TRUE] -> w305
          frame "ASCII", Default {
          }
          frame "Enter", "Return" {
          }
        }
        n162 = case shown="9" w306 {
          tunnel: [FALSE TRUE] -> w304
          frame 0, Default {
          }
          frame 9 {
            # "TAB"
          }
        }
        n163 = Or(x=w305, y=w304) -> (x .or. y?=w303:bool)
        n164 = case shown="True" w303 {
          tunnel: w308 -> [_ w318]
          frame False {
          }
          frame True {
            n165 = property on="Property Node" class="MCListbox (strict)"(reference=w318) -> (reference out=w317:refnum<vi>, "ActiveCell"=w313:T2)  [unwired: 1 in, 1 out]
            "Active Cell:Active Cell" <- w313
            n166 = Unbundle By Name(w313) -> ("Row"=w316:i32, "Column"=w315:i32)
            n167 = Increment(x=w316) -> (x+1=w314:i32)
            n168 = while {
              tunnel: w317 -> [w348]
              tunnel: w315 -> [w342]
              tunnel: w314 -> [w321]
              tunnel: w313 -> [w333]
              i -> [w336]
              stop <- w334 stop-if-true
              # "Exit on 1st Valid Cell Found or No\nMore Cells Left"
              n169 = local read "# of Columns in DB Table"() -> (w323:i32)
              n170 = Add(x=w321, y=w336) -> (x+y=w327:i32)
              n171 = Bundle By Name(cluster=w333, "Row"=w327) -> (w332:T2)
              n172 = property class="MCListbox (strict)"(reference=w348) -> ("ItemNames"=w349:string[][])  [unwired: 1 in, 2 out]
              n173 = Subtract(x=w323, y=1) -> (x-y=w324:i32)
              n174 = Index Array(array=w349, index (row) #1=w327, index (col) #1=DB_-_Config_Table_Enum."Type" ("Data Type"), index (row) #2=w327, index (col) #2=DB_-_Config_Table_Enum."Column Name" ("Column Name"), index (row) #3=w327, index (col) #3=DB_-_Config_Table_Enum."Description" ("Column Name")) -> (element #1=w351:string, element #2=w338:string, element #3=w325:string)
              n175 = Greater Or Equal?(x=w321, y=w324) -> (x >= y?=w320:bool)
              n176 = local read "Foreign Keys"() -> (w340:string[])
              n177 = local read "IDENTITY COLUMN"() -> (w350:string)
              n178 = To Upper Case(1:w325) -> (0:w331:string)
              n179 = Match Pattern(string=w331, regular expression="(AUTO)") -> (offset past match=w329:i32)  [unwired: 1 in, 3 out]
              n180 = Search 1D Array "isNOTForeignKey?"(1D array=w340, element=w338) -> (index of element=w339:i32)  [unwired: 1 in]
              n181 = Match Pattern(string=w351, regular expression="varbinary" ("y")) -> (offset past match=w353:i32)  [unwired: 1 in, 3 out]
              n182 = Not Equal? "Column Name not Inactive"(x=w338, y="Inactive") -> (x != y?=w345:bool)
              n183 = Not Equal? "isNOTIdentity"(x=w338, y=w350) -> (x != y?=w344:bool)
              n184 = Less Than 0? "isNOT(AUTO)"(x=w329) -> (x < 0?=w328:bool)
              n185 = Not "isNotLastRow"(x=w320) -> (.not. x?=w319:bool)
              n186 = Less Than 0?(x=w339) -> (x < 0?=w337:bool)
              n187 = Less Than 0? "NOTvarbinary"(x=w353) -> (x < 0?=w346:bool)
              n188 = Equal? "isDataColumn"(x=w342, y=DB_-_Config_Table_Enum."Value (Data)" ("Data Column")) -> (x = y?=w341:bool)
              n189 = Compound Arithmetic op=AND(w346, w345, w344, w341, w328, w337, w319) -> (w335:bool)
              n190 = case shown="True" w335 {
                tunnel: w332 -> [_ w362]
                tunnel: w348 -> [w356 w361]
                tunnel: w327 -> [_ w360]
                frame False {
                  n191 = disable-structure shown="Disabled" {
                    disable-tunnel: w356 -> [w359 _]
                    frame Disabled {
                      n192 = property on="Property Node" class="MCListbox (strict)"(reference=w359, "EditPos"=T2 {"Row"=-2, "Column"=-2} ("Edit Position"), "Value"=-1) -> ()  [unwired: 1 in, 2 out]
                    }
                    frame Enabled {
                    }
                  }
                }
                frame True {
                  # "Next Valid Cell"
                  n193 = property on="Property Node" class="MCListbox (strict)"(reference=w361, "ActiveCell"=w362, "EditPos"=w362, "Value"=w360) -> ()  [unwired: 1 in, 2 out]
                }
              }
              n194 = Or(x=w335, y=w320) -> (x .or. y?=w334:bool)
            }
          }
        }
      }
      event "Multicolumn Listbox": Mouse Down {
        w381 = 1  # Left Mouse Click
        # "Check if Cell is Valid"
        # "Get Clicked Col Hdr cannot\nbe captured here so we have\nto use Point To Row Column"
        n195 = event-data() -> ("Time"=w380:u32, "CtlRef"=w379:refnum<vi>, "Coords"=w378:T16, "Button"=w377:u16)  [unwired: 1 in, 4 out]
        n196 = property on="Property Node" class="CmbBox"(reference=w376, "Visible"=FALSE) -> (reference out=w393:refnum<vi>)  [unwired: 1 in, 1 out]
        n197 = invoke class="MCListbox (strict)" method="Point To Row Column"(reference=w379, "Point"=w378) -> (reference out=w390:refnum<vi>, "InBounds"=w387:bool, "CellPosition"=w392:T2)  [unwired: 5 in, 4 out]
        n198 = property class="MCListbox (strict)"(reference=w390) -> (reference out=w389:refnum<vi>, "ItemNames"=w374:string[][], "ColHdrString"=w383:string[])  [unwired: 1 in, 1 out]
        n199 = Unbundle By Name(w392) -> ("Row"=w375:i32, "Column"=w373:i32)
        n200 = Index Array(array=w383, index=w373) -> (element=w364:string)
        n201 = local read "Foreign Keys"() -> (w372:string[])
        n202 = Index Array(array=w374, index (row)=w375, index (col)=DB_-_Config_Table_Enum."Column Name" ("Column Name")) -> (element=w371:string)
        "Foreign Key Selected" <- w371
        n203 = Search 1D Array "isForeignKey?"(1D array=w372, element=w371) -> (index of element=w370:i32)  [unwired: 1 in]
        n204 = Equal? "isDataColumn"(x=w373, y=DB_-_Config_Table_Enum."Value (Data)" ("Data Column")) -> (x = y?=w388:bool)
        n205 = Equal?(x=w377, y=w381) -> (x = y?=w382:bool)
        n206 = Greater Or Equal To 0?(x=w370) -> (x >= 0?=w363:bool)
        n207 = Compound Arithmetic op=AND(w363, w388) -> (w386:bool)
        n208 = property class="MCListbox (strict)"(reference=w389, "ActiveCell"=w392) -> (reference out=w391:refnum<vi>)  [unwired: 1 in, 1 out]
        n209 = And(x=w386, y=w387) -> (x .and. y?=w384:bool)
        n210 = And(x=w384, y=w382) -> (x .and. y?=w365:bool)
        n211 = case shown="True" w365 {
          tunnel: w392 -> [w418 w444]
          tunnel: w393 -> [_ w443]
          tunnel: w391 -> [w417 w442]
          tunnel: w375 -> [_ w441]
          tunnel: w386 -> [_ _]
          tunnel: w364 -> [_ w440]
          tunnel: w380 -> [_ w439]
          tunnel: w378 -> [_ w438]
          tunnel: w367 -> [_ w437]
          tunnel: w366 -> [_ w436]
          frame False {
            # "Scroll Bar is clicked OR \nNOT Foreign Key Celll is clicked"
            n212 = Unbundle By Name(w418) -> ("Row"=w399:i32, "Column"=w406:i32)
            n213 = property class="MCListbox (strict)"(reference=w417) -> ("ItemNames"=w416:string[][])  [unwired: 1 in, 2 out]
            n214 = Index Array(array=w416, index (row) #1=w399, index (col) #1=DB_-_Config_Table_Enum."Type" ("Data Type"), index (row) #2=w399, index (col) #2=DB_-_Config_Table_Enum."Column Name" ("Column Name"), index (row) #3=w399, index (col) #3=DB_-_Config_Table_Enum."Description" ("Column Name")) -> (element #1=w411:string, element #2=w403:string, element #3=w398:string)
            n215 = local read "IDENTITY COLUMN"() -> (w412:string)
            n216 = To Upper Case(1:w398) -> (0:w397:string)
            n217 = Match Pattern(string=w397, regular expression="(AUTO)") -> (offset past match=w395:i32)  [unwired: 1 in, 3 out]
            n218 = Match Pattern(string=w411, regular expression="varbinary" ("y")) -> (offset past match=w409:i32)  [unwired: 1 in, 3 out]
            n219 = Not Equal? "Column Name not Inactive"(x=w403, y="Inactive") -> (x != y?=w404:bool)
            n220 = Not Equal? "isNOTIdentity"(x=w403, y=w412) -> (x != y?=w405:bool)
            n221 = Less Than 0? "isNOT(AUTO)"(x=w395) -> (x < 0?=w394:bool)
            n222 = Equal? "isDataColumn"(x=w406, y=DB_-_Config_Table_Enum."Value (Data)" ("Data Column")) -> (x = y?=w413:bool)
            n223 = Less Than 0? "NOTvarbinary"(x=w409) -> (x < 0?=w408:bool)
            n224 = Compound Arithmetic op=AND(w408, w404, w405, w413, w394) -> (w407:bool)
            n225 = case shown="True" w407 {
              tunnel: w417 -> [w433 w435]
              tunnel: w418 -> [w424 _]
              frame True {
                # "Storing ActiveCell and EditPos does not seem to work"
                # "Editable Row is clicked.\nNOT Foreign Key"
                n226 = property class="MCListbox (strict)"(reference=w433) -> (reference out=w432:refnum<vi>, "RowHdrs[]"=w431:string[], "ItemNames"=w425:string[][])  [unwired: 1 in, 1 out]
                n227 = Unbundle By Name(w424) -> ("Row"=w423:i32, "Column"=w422:i32)
                n228 = Cluster To Array(cluster=w424) -> (array=w430:i32[])
                n229 = Array To Spreadsheet String(delimiter (Tab)=",", array=w430, 3:"" ("format string")) -> (spreadsheet string=w428:string)
                n230 = Index Array(array=w425, index (row)=w423, index (col)=w422) -> (element=w421:string)
                n231 = Replace Array Subset(array=w431, new element #1=w428, index #1=MCListbox_-_Enum."Initial (KD?)" ("MCListbox Enum"), new element #2=w421, index #2=MCListbox_-_Enum."Initial Text" ("MCListbox Enum")) -> (w427:string[])
                n232 = property class="MCListbox (strict)"(reference=w432, "RowHdrs[]"=w427) -> ()  [unwired: 1 in, 2 out]
              }
              frame False {
                # "If set -2.-2 to EditPostion, row 0 column -1 will be set - dunno why\nSo we use KeyFocus instead."
                # "Invalid Cell"
                n233 = property class="MCListbox (strict)"(reference=w435, "Key Focus"=FALSE) -> ()  [unwired: 1 in, 2 out]
              }
            }
          }
          frame True {
            # "Inbound - Selection is Col Hdrs OR (Data Column AND Foreign KEY)"
            n234 = case shown="0.." w441 {
              tunnel: w444 -> [w484 _]
              tunnel: w442 -> [w483 _]
              tunnel: w443 -> [w482 _]
              tunnel: w440 -> [_ _]
              tunnel: w439 -> [_ _]
              tunnel: w438 -> [_ _]
              tunnel: w437 -> [w464 _]
              tunnel: w436 -> [w463 _]
              frame 0.. {
                # "Updates ComboBox Strings[]"
                # "Get referenced _table"
                # "Get referenced column"
                # "Get row"
                # "Row 0 and above is selected, NOT Col Hdrs\nChange Position, Size, Color and Strings[] of CmbBox"
                n235 = call "MCListbox - Move Combo Box.vi"("CellPosition"=w484, "Combo Box in"=w482, "MulticolumnListbox in"=w483) -> ("Combo Box out"=w462:refnum<vi>)  [unwired: 7 in, 1 out]
                n236 = local read "Table Name"() -> (w456:T4)
                n237 = local read "Foreign Key Selected"() -> (w480:string)
                n238 = call "DB - Get Foreign Keys References.vi"("error in (no error)"=w463, "Select"=T14."Find FK's Primary Schema.Table", "DB.Schema.Table"=w456, "connection reference"=w464) -> ("error out"=w475:errorcluster, "Foreign Keys References"=w478:string[][], "connection reference"=w476:T11)  [unwired: 5 in]
                n239 = Index Array(array=w478, index (col)=6 ("disabled index (col)")) -> (element=w479:string[])  [unwired: 1 in]
                n240 = Search 1D Array(1D array=w479, element=w480) -> (index of element=w458:i32)  [unwired: 1 in]
                n241 = Index Array(array=w478, index (row) #1=w458, index (col) #1=6 ("index"), index (row) #2=w458, index (col) #2=4 ("disabled index (col)"), index (row) #3=w458, index (col) #3=5 ("disabled index (col)")) -> (element #1=w448:string, element #2=w447:string, element #3=w446:string)
                n242 = Search and Replace String(replace all?=TRUE ("replace all? (F)"), input string="SELECT [<A>] FROM [<Schema>].[<Table>]\nGROUP BY [<A>]\nORDER BY [<A>]", search string="<A>", replace string=w448) -> (result string=w452:string)  [unwired: 4 in, 3 out]
                n243 = Search and Replace String(input string=w452, search string="<Schema>", replace string=w447) -> (result string=w450:string)  [unwired: 5 in, 3 out]
                n244 = Search and Replace String(input string=w450, search string="<Table>", replace string=w446) -> (result string=w445:string)  [unwired: 5 in, 3 out]
                n245 = call-poly <vilib>:"DB Tools Execute Query.vi"("error in (no error)"=w475, "SQL query"=w445, "connection reference"=w476) -> ("error out"=w474:errorcluster, "recordset reference"=w473:T17)  [unwired: 5 in]
                n246 = call-poly <vilib>:"DB Tools Fetch Recordset Data.vi"("error in (no error)"=w474, "recordset reference"=w473) -> ("error out"=w470:errorcluster, "recordset data"=w471:variant[][], "recordset reference out"=w472:T17)  [unwired: 3 in]
                n247 = xnode "Database Variant To Data"("database variant"=w471, "error in (no error)"=w470, "type"=string[][] []) -> ("data"=w467:string[][], "error out"=w469:errorcluster)
                n248 = call-poly <vilib>:"DB Tools Free Object.vi"("error in (no error)"=w469, "recordset reference"=w472) -> ("error out"=w457:errorcluster)  [unwired: 8 in, 1 out]
                n249 = Index Array(array=w467, index (col)=0 ("index (row)")) -> (element=w466:string[])  [unwired: 1 in]
                n250 = global write "Global SRTRS.vi" "DB Error"(w457) -> ()
                n251 = property class="CmbBox"(reference=w462, "Strings[]"=w466) -> ()  [unwired: 1 in, 2 out]
              }
              frame Default {
                # "Col Hdr"
              }
            }
          }
        }
      }
      event "Select Foreign Key": Mouse Leave {
        n252 = event-data() -> ()  [unwired: 1 in, 4 out]
        n253 = property on="Select Foreign Key" class="CmbBox"("Visible"=FALSE) -> ()  [unwired: 2 in, 2 out]
      }
      event "Multicolumn Listbox": Edit Cell; "Extra Event From \"Select Foreign Key\"": Value Change {
        # "2014-09-17\n       0           |           1           |          2           |      3         |     4\nCol Name  |  Description  |  Value Type  |  Length   | Value \n(Fieldname)                          (Data Type)                    (Data)\n                                                                                     DataColumn"
        # "update  dbo.Table_Order \nSet OrderNo='105',OperationNo=105,NCRNo='A123',CustomerName='A111' \nwhere dbo.Table_Order.OrderNo = 105"
        # "Columns\nValue\nType \nLength"
        n254 = event-data() -> ("Type"=→"Type":T3, "Time"=→"MCListBox EditCell, Extra Event From  \"Select Foreign Key\"":u32)  [unwired: 1 in, 2 out]
        n255 = property class="MCListbox (strict)" props=["EditPos", "ItemNames", "RowHdrs[]"](reference=w535) -> (reference out=w555:refnum<vi>, error out=w554:errorcluster, "ItemNames"=w544:string[][], "RowHdrs[]"=w553:string[])  [unwired: 1 in, 1 out]
        n256 = local write "Extra Event From \"Select Foreign Key\""(FALSE ("Extended Event From \"Select Foreign Key Value Changed\"")) -> ()
        n257 = Index Array(array=w553, index #1=MCListbox_-_Enum."Initial (KD?)" ("MCListbox Enum"), index #2=MCListbox_-_Enum."Initial Text" ("MCListbox Enum")) -> (element #1=w552:string, element #2=w541:string)
        n258 = Spreadsheet String To Array(delimiter (Tab)=",", format string="", spreadsheet string=w552, array type (2D Dbl)=i32[] []) -> (array=w549:i32[])
        n259 = Index Array(array=w549) -> (element #1=w548:i32, element #2=w536:i32)  [unwired: 2 in]
        n260 = Index Array(array=w544, index (row)=w548) -> (element=w557:string[])  [unwired: 1 in]
        n261 = Index Array(array=w557, index #1=0 ("index")) -> (element #1=w542:string, element #3=w556:string, element #4=w546:string, element #5=w531:string)  [unwired: 4 in, 1 out]
        n262 = case "Type" shown="\"bit\"" w556 {
          tunnel: w531 -> [w560 w563 w570 w572 w576]
          tunnel: w542 -> [_ _ _ _ _]
          tunnel: w546 -> [_ w562 w566 _ _]
          tunnel: [w560 w561 w565 w571 w573] -> w545
          frame "False", Default {
          }
          frame "char", "nchar", "nvarchar", "varchar" {
            n263 = Decimal String To Number(string=w562) -> (number=w564:i32)  [unwired: 2 in, 1 out]
            n264 = Search/Split String(string=w563, offset (0)=w564) -> (substring before match=w561:string)  [unwired: 1 in, 2 out]
          }
          frame "int" {
            n265 = Decimal String To Number(string=w570) -> (number=w569:i32)  [unwired: 2 in, 1 out]
            n266 = Decimal String To Number(string=w566) -> (number=w568:i32)  [unwired: 2 in, 1 out]
            n267 = Number To Decimal String(number=w569) -> (decimal integer string=w567:string)  [unwired: 1 in]
            n268 = Search/Split String(string=w567, offset (0)=w568) -> (substring before match=w565:string)  [unwired: 1 in, 2 out]
          }
          frame "datetime" {
            # "2014-08-02 21:54:05"
            n269 = call "String - Convert String Only TimeStamp II.vi"("YYYY-mm-dd HH:MM:SS"=w572) -> ("YYYY-mm-dd HH:MM:SS"=w571:string)  [unwired: 9 in, 1 out]
          }
          frame "bit" {
            n270 = String Subset(string=w576, length (rest)=1 ("length (rest)")) -> (substring=w574:string)  [unwired: 1 in]
            n271 = case shown="\"1\", \"T\", \"t\"" w574 {
              selector: w574 -> [_ w578]
              tunnel: ["0" w578] -> w573
              frame "0", Default {
              }
              frame "1", "T", "t" {
              }
            }
          }
        }
        n272 = Not Equal?(x=w545, y=w541) -> (x != y?=w532:bool)
        n273 = Replace Array Subset(array=w544, new element=w545, index (row)=w548, index (col)=w536) -> (w543:string[][])
        n274 = local write "Changed"(w532) -> ()
        n275 = property class="MCListbox (strict)"(reference=w555, error in=w554, "ItemNames"=w543) -> ()  [unwired: 2 out]
        n276 = case shown="False" w532 {
          tunnel: [T9."Disabled and Grayed Out" ("Disabled") T9."Enabled" ("Disabled")] -> w533
          frame False {
          }
          frame True {
          }
        }
        n277 = property on="Save" class="Bool"("DisabledEnum"=w533) -> ()  [unwired: 2 in, 2 out]
      }
      event "Save", "Delete": Value Change {
        # "2014-09-17\n       0           |           1           |          2           |      3         |     4\nCol Name  |  Description  |  Value Type  |  Length   | Value \n(Fieldname)                          (Data Type)                    (Data)\n                                                                                     DataColumn"
        # "Error when no updateable Columns"
        # "USE [SRTRS]\nGO\n\nINSERT INTO [MasterData].[Material]\n           ([MaterialNo]\n           ,[Revision]\n           ,[Description]\n           ,[ImageFile]\n           ,[Inactive])\n     VALUES\n           (<MaterialNo,>\n           ,<Revision>\n           ,<Description,>\n           ,<ImageFile>\n           ,<Inactive>)\nGO"
        # "USE [<DB>]\n\nUPDATE [<Schema>].[<Table>]\nSET <AB>\nWHERE <C>"
        n278 = event-data() -> ("CtlRef"=w603:refnum<vi>)  [unwired: 1 in, 5 out]
        n279 = property class="Bool"(reference=w603) -> (reference out=w597:refnum<vi>, "Label.Text"=w580:string)  [unwired: 1 in, 1 out]
        n280 = local write "Changed"(FALSE ("Changed")) -> ()
        n281 = property on="Multicolumn Listbox" class="MCListbox (strict)"() -> ("ItemNames"=w612:string[][])  [unwired: 2 in, 2 out]
        n282 = local read "Primary Keys"() -> (w604:string[])
        n283 = case shown="\"Delete\", Default" w580 {
          tunnel: w612 -> [_ w673]
          tunnel: [w659 w670] -> w585
          tunnel: [w657 w669] -> w596
          tunnel: w604 -> [_ w668]
          tunnel: [w656 TRUE ("T button?")] -> w598
          tunnel: w597 -> [_ w663]
          frame "Delete", Default {
            # "Delete NOT Greyed out here.\nWill be checked at the End of Transaction"
            # "Set Inactive = 1"
            n284 = local read "Application"() -> (w652:string)
            n285 = call "Msgbox - Message Handler.vi"("Application (Default SRTRS)"=w652, "Short Description (When DB Not Available)"="Delete Record", "Description (When DB Not Available)"="Current record will be deleted. Do you want to proceed?", "<.?....> Message Code"="<W 704>") -> ("MHandler Error"=w651:errorcluster, "OK Out"=w656:bool)  [unwired: 5 in, 1 out]
            n286 = local write "MHandler"(w651) -> ()
            n287 = Build Array("Inactive") -> (w659:string[])
            n288 = Build Array("1") -> (w657:string[])
          }
          frame "Save" {
            n289 = Index Array(array=w673, index (col) #1=DB_-_Config_Table_Enum."Column Name" ("COLUMN NAMES"), index (col) #2=DB_-_Config_Table_Enum."Value (Data)" ("VALUES"), index (col) #3=DB_-_Config_Table_Enum."Type" ("TYPE")) -> (element #1=w671:string[], element #2=w666:string[], element #3=w664:string[])  [unwired: 3 in]
            n290 = property on="Property Node" class="Bool"(reference=w663, "DisabledEnum"=T9."Disabled and Grayed Out" ("Disabled")) -> ()  [unwired: 1 in, 2 out]
            n291 = for {
              tunnel: w671 -> [w678] mode=indexing
              tunnel: [w678] -> w670 mode=indexing if=w681
              tunnel: w666 -> [w684] mode=indexing
              tunnel: [w684] -> w669 mode=indexing if=w681
              tunnel: w668 -> [w683]
              tunnel: w664 -> [w677] mode=indexing
              # "Should we Insert our own Primary Keys?"
              # "Get all Update-able Column Names"
              n292 = local read "IDENTITY COLUMN"() -> (w679:string)
              n293 = Search 1D Array(1D array=w683, element=w678) -> (index of element=w682:i32)  [unwired: 1 in]
              n294 = Not Equal? "IsNotVarBinary"(x=w677, y="varbinary") -> (x != y?=w676:bool)
              n295 = Less Than 0? "IsNotPrimaryKeys"(x=w682) -> ()  [unwired: 1 out]
              n296 = Not Equal? "IsNotIdentity"(x=w678, y=w679) -> (x != y?=w680:bool)
              n297 = Compound Arithmetic op=AND(TRUE ("value"), w680, w676) -> (w681:bool)
            }
          }
        }
        n298 = Index Array(array=w612, index (col)=0 ("disabled index (col)")) -> (element=w613:string[])  [unwired: 1 in]
        n299 = property on="Table Name" class="CmbBox (strict)"() -> ("Value"=w599:T4)  [unwired: 2 in, 2 out]
        n300 = for {
          tunnel: w604 -> [w696] mode=indexing
          tunnel: w613 -> [w700]
          tunnel: w612 -> [w698]
          shift-right: [w690] -> w605
          shift-left: "" -> [w685]
          i -> [w691]
          w688 = " AND "  # add 'AND' if more  than 1 Primary Key
          # "Get Primary Key(s) Values"
          n301 = Greater Than 0?(x=w691) -> (x > 0?=w689:bool)
          n302 = Search 1D Array(1D array=w700, element=w696) -> (index of element=w699:i32)  [unwired: 1 in]
          n303 = Index Array(array=w698, index (row)=w699, index (col)=DB_-_Config_Table_Enum."Value (Data)" ("VALUES")) -> (element=w693:string)
          n304 = Select(t=w688, s=w689, f="") -> (s? t:f=w686:string)
          n305 = Concatenate Strings(w685, w686, w696, " = " ("string"), "'" ("string"), w693, "'" ("string")) -> (w690:string)
        }
        n306 = for {
          tunnel: w596 -> [w705] mode=indexing
          shift-right: [w702] -> w616
          shift-left: "" -> [w704]
          tunnel: w585 -> [w701] mode=indexing
          n307 = Search and Replace String(input string=",<A> = '<B>' ", search string="<A>", replace string=w701) -> (result string=w707:string)  [unwired: 5 in, 3 out]
          n308 = Search and Replace String(input string=w707, search string="<B>", replace string=w705) -> (result string=w703:string)  [unwired: 5 in, 3 out]
          n309 = Concatenate Strings(w704, w703) -> (w702:string)
        }
        n310 = call "DB - Split DB.Schema.Table.vi"("DB.Schema.Table"=w599) -> ("DB.Schema.Table"=w583:T18)  [unwired: 10 in]
        n311 = Search/Split String "Skip 1st ,"(string=w616, offset (0)=1) -> (match + rest of string=w608:string)  [unwired: 1 in, 2 out]
        n312 = call "DB - Replace DB.Schema.Table.vi"("DB.Schema.Table"=w583, "string in"="USE [<DB>]\n\nUPDATE [<Schema>].[<Table>]\nSET <AB>\nWHERE <C>\n ") -> ("string out"=w610:string)  [unwired: 8 in, 1 out]
        n313 = Search and Replace String(input string=w610, search string="<AB>", replace string=w608) -> (result string=w607:string)  [unwired: 5 in, 3 out]
        n314 = Search and Replace String(input string=w607, search string="<C>", replace string=w605) -> (result string=w589:string)  [unwired: 5 in, 3 out]
        n315 = call "DB - Replace DB.Schema.Table.vi"("DB.Schema.Table"=w583, "string in"="USE [<DB>]\n\nINSERT INTO [<Schema>].[<Table>]\n( <A>)\nVALUES\n( <B>)\n ") -> ("string out"=w584:string)  [unwired: 8 in, 1 out]
        n316 = call "DB - Array to Columns.vi"("Array"=w585) -> ("[Columns]"=w594:string)  [unwired: 10 in]
        n317 = local read "New Record in UI not in DB"() -> (w590:bool)
        n318 = Search and Replace String(input string=w584, search string="<A>", replace string=w594) -> (result string=w591:string)  [unwired: 5 in, 3 out]
        n319 = call "DB - Array to Values.vi"("Array (0xFFFE autodetect)"=w596) -> ("<Values>"=w593:string)  [unwired: 10 in]
        n320 = Search and Replace String(input string=w591, search string="<B>", replace string=w593) -> (result string=w588:string)  [unwired: 5 in, 3 out]
        n321 = Select(t=w588, s=w590, f=w589) -> (s? t:f=w587:string)
        "SQL Query" <- w587
        n322 = case shown="True" w598 {
          tunnel: w619 -> [_ w650]
          tunnel: w587 -> [_ w649]
          tunnel: [_ w648] -> w581
          tunnel: w580 -> [_ w645]
          tunnel: ["" w645] -> w579
          frame False {
          }
          frame True {
            n323 = call-poly <vilib>:"DB Tools Execute Query.vi"("SQL query"=w649, "connection reference"=w650) -> ("error out"=w646:errorcluster, "recordset reference"=w647:T17)  [unwired: 6 in]
            n324 = call-poly <vilib>:"DB Tools Free Object.vi"("error in (no error)"=w646, "recordset reference"=w647) -> ("error out"=w648:errorcluster)  [unwired: 8 in, 1 out]
          }
        }
        "DB" <- w581
        n325 = global write "Global SRTRS.vi" "DB Error"(w581) -> ()
        n326 = case shown="\"Delete\"" w579 {
          tunnel: w581 -> [w622 w633]
          frame "Save", Default {
            n327 = case shown="No Error" w622 {
              tunnel: ["Record Save" ("Short Description (When DB Not Available)") "Save Record Fail" ("Short Description (When DB Not Available)")] -> w625
              tunnel: ["Record saved successfully." ("{Save .....} [.....] =") "Please retry with valid datatype and length." ("{Save .....} [.....] =")] -> w624
              tunnel: ["<I 705>" ("<.?....> Message Code") "<E 706>" ("<.?....> Message Code")] -> w623
              frame No Error {
                n328 = disable-structure shown="Disabled" {
                  frame Disabled {
                    n329 = property on="Table Name" class="CmbBox (strict)" props=["Value"]() -> ()  [unwired: 2 in, 3 out]
                  }
                  frame Enabled {
                  }
                }
              }
              frame Error {
              }
            }
            n330 = local write "New Record in UI not in DB"(FALSE ("New Record in UI not in DB")) -> ()
            n331 = local read "Application"() -> (w620:string)
            n332 = call "Msgbox - Message Handler.vi"("Application (Default SRTRS)"=w620, "Short Description (When DB Not Available)"=w625, "Description (When DB Not Available)"=w624, "<.?....> Message Code"=w623) -> ("MHandler Error"=w621:errorcluster)  [unwired: 5 in, 2 out]
            n333 = local write "MHandler"(w621) -> ()
          }
          frame "Delete" {
            n334 = local read "Include Inactive"() -> (w634:bool)
            n335 = disable-structure shown="Disabled" {
              frame Disabled {
                n336 = property on="Table Name" class="CmbBox (strict)" props=["Value"]() -> ()  [unwired: 2 in, 3 out]
              }
              frame Enabled {
              }
            }
            n337 = case shown="False" w634 {
              frame False {
                # "- 1 record"
                n338 = local read "Record Count"() -> (w642:i32)
                n339 = Decrement(x=w642) -> (x-1=w641:i32)
                n340 = local write "Record Count"(w641) -> ()
                n341 = Equal To 0?(x=w641) -> (x = 0?=w640:bool)
                n342 = case shown="True" w640 {
                  frame False {
                  }
                  frame True {
                    # "Refresh Table since NO record left"
                    n343 = property on="Table Name" class="CmbBox (strict)"() -> ("Value"=w643:T4)  [unwired: 2 in, 2 out]
                    n344 = property on="Table Name" class="CmbBox (strict)"("Val(Sgnl)"=w643) -> ()  [unwired: 2 in, 2 out]
                  }
                }
              }
              frame True {
                # "No Change"
              }
            }
            n345 = case shown="Error" w633 {
              frame No Error {
              }
              frame Error {
                n346 = local read "Application"() -> (w636:string)
                n347 = call "Msgbox - Message Handler.vi"("Application (Default SRTRS)"=w636, "Short Description (When DB Not Available)"="Delete Record Failed.", "Description (When DB Not Available)"="Record cannot be deleted.", "<.?....> Message Code"="<E 707>") -> ("MHandler Error"=w635:errorcluster)  [unwired: 5 in, 2 out]
                n348 = local write "MHandler"(w635) -> ()
              }
            }
          }
        }
        n349 = property on="Current Record" class="DigNum (strict)"(error in=w581) -> (error out=w601:errorcluster, "Value"=w600:i32)  [unwired: 1 in, 1 out]
        n350 = property on="Current Record" class="DigNum (strict)"(error in=w601, "Val(Sgnl)"=w600) -> (error out=w582:errorcluster)  [unwired: 1 in, 1 out]
        n351 = local write "Property Node"(w582) -> ()
      }
      event "Database Group": Mouse Down? {
        n352 = event-data() -> ()  [unwired: 1 in, 8 out]
        n353 = local read "Application"() -> (w710:string)
        n354 = local read "DB.Config.TableGroupType"() -> (w714:string)
        n355 = local read "DB.Config.TableGroup"() -> (w713:string)
        n356 = call "DB - [Config].[TableGroup].vi"("Application"=w710, "Table Group Enum"=DB_-_Table_Group_Enum."SELECT [Description]", "DB.Config.TableGroup"=w713, "DB.Config.TableGroupType"=w714) -> ("SUMMARY"=w711:errorcluster, "data"=w718:string[])  [unwired: 5 in, 1 out]
        n357 = local write "DB"(w711) -> ()
        n358 = property on="Database Group" class="CmbBox"("Strings[]"=w718) -> (error out=w716:errorcluster, "Value"=w715:string)  [unwired: 2 in, 1 out]
        n359 = property on="Database Group" class="CmbBox"(error in=w716, "Val(Sgnl)"=w715) -> (error out=w712:errorcluster)  [unwired: 1 in, 1 out]
        n360 = local write "Property Node"(w712) -> ()
        n361 = event-data() -> ()  [unwired: 2 in, 1 out]
      }
      event "New", "Copy": Value Change {
        n362 = event-data() -> ("CtlRef"=w726:refnum<vi>)  [unwired: 1 in, 5 out]
        n363 = case shown="False" "New" {
          tunnel: ["<W 702>" ("<.?....> Message Code") "<W 703>" ("<.?....> Message Code")] -> w725
          tunnel: ["Create New Record" ("Short Description (When DB Not Available)") "Copy Record" ("Short Description (When DB Not Available)")] -> w724
          tunnel: ["All unsaved data will be lost. Do you want to proceed?" ("Description (When DB Not Available)") "All current data except bold fields will be copied to new record. Do you want to proceed?" ("Description (When DB Not Available)")] -> w723
          frame True {
            # "New is clicked"
          }
          frame False {
            # "Copy is clicked"
          }
        }
        n364 = local read "Application"() -> (w719:string)
        n365 = call "Msgbox - Message Handler.vi"("Application (Default SRTRS)"=w719, "Short Description (When DB Not Available)"=w724, "Description (When DB Not Available)"=w723, "<.?....> Message Code"=w725) -> ("MHandler Error"=→"MHandler":errorcluster, "OK Out"=w722:bool)  [unwired: 5 in, 1 out]
        n366 = case shown="True" w722 {
          tunnel: w727 -> [_ w753]
          tunnel: w726 -> [_ w738]
          frame False {
          }
          frame True {
            w749 = DB_-_Config_Table_Enum."Value (Data)" ("Values")
            # "Fieldname         | Description | DataType | Length  | Record \nColumn Name | Description |     Type      | Length | Value (Data)"
            # "New:\nAdd Record Count\nClears All Data Fields\nSet \"New Record in UI not in DB\" Flag\n\nCopy:\nAdd Record Count\nClears ONLY Primary & Foreign Keys Fields\nSet \"New Record in UI not in DB\" Flag"
            n367 = property on="Property Node" class="MCListbox (strict)"(reference=w753) -> (reference out=w750:refnum<vi>, "ItemNames"=w751:string[][])  [unwired: 1 in, 1 out]
            n368 = local read "New Record in UI not in DB"() -> (w734:bool)
            n369 = property class="Bool"(reference=w738) -> ("Label.Text"=w737:string)  [unwired: 1 in, 2 out]
            n370 = local read "Foreign Keys"() -> (w740:string[])
            n371 = local read "Primary Keys"() -> (w741:string[])
            n372 = Index Array(array=w751, index (col) #1=w749, index (col) #2=DB_-_Config_Table_Enum."Column Name" ("Values"), index (col) #3=DB_-_Config_Table_Enum."Type" ("Values")) -> (element #1=w752:string[], element #2=w748:string[], element #3=w742:string[])  [unwired: 3 in]
            n373 = Equal?(x=w737, y="Copy") -> (x = y?=w735:bool)
            n374 = Build Array (concatenate)(w741, w740) -> (w739:string[])
            n375 = case shown="False" w734 {
              frame False {
                n376 = local read "Record Count"() -> (w755:i32)
                n377 = local write "New Record in UI not in DB"(TRUE ("New Record in UI not in DB")) -> ()
                n378 = Increment(x=w755) -> (x+1=w756:i32)
                n379 = local write "Record Count"(w756) -> ()
                n380 = property on="Current Record" class="DigNum (strict)"("Value"=w756) -> ()  [unwired: 2 in, 2 out]
              }
              frame True {
                # "New Record NOT saved in DB\nSo we do not increase Displayed Record Count"
              }
            }
            n381 = for {
              tunnel: w752 -> [w757] mode=indexing
              tunnel: w748 -> [w763] mode=indexing
              tunnel: [w765] -> w747 mode=indexing
              tunnel: w742 -> [w764] mode=indexing
              tunnel: w739 -> [w762]
              tunnel: w735 -> [w759]
              n382 = Search 1D Array(1D array=w762, element=w763) -> (index of element=w761:i32)  [unwired: 1 in]
              n383 = Less Than 0?(x=w761) -> (x < 0?=w760:bool)
              n384 = And "Copy AND NOT Primary/Foreign Key"(x=w760, y=w759) -> (x .and. y?=w758:bool)
              n385 = case shown="\"False\", Default" w763 {
                tunnel: [w769 "0"] -> w765
                tunnel: w764 -> [w768 _]
                tunnel: w758 -> [w767 _]
                tunnel: w757 -> [w766 _]
                frame "False", Default {
                  n386 = case shown="\"varbinary\"" w768 {
                    tunnel: ["<Binary data>" w771] -> w769
                    tunnel: w767 -> [_ w774]
                    tunnel: w766 -> [_ w773]
                    frame "varbinary" {
                      # "Always assign <Binary data>"
                    }
                    frame "", Default {
                      # "Either COPY or CLEAR"
                      n387 = Select(t=w773, s=w774, f="") -> (s? t:f=w771:string)
                    }
                  }
                }
                frame "Inactive" {
                }
              }
            }
            n388 = property on="Delete" class="Bool"("DisabledEnum"=T9."Disabled and Grayed Out" ("Disabled")) -> ()  [unwired: 2 in, 2 out]
            n389 = Replace Array Subset(array=w751, new element=w747, index (col)=w749) -> (w746:string[][])  [unwired: 1 in]
            n390 = property on="Property Node" class="MCListbox (strict)"(reference=w750, "ItemNames"=w746) -> ()  [unwired: 1 in, 2 out]
          }
        }
      }
      event "Select Foreign Key": Value Change {
        n391 = event-data() -> ()  [unwired: 1 in, 6 out]
        n392 = property class="CmbBox"(reference=w781, "Visible"=FALSE) -> ("Desc"=w778:string, "Value"=w777:string)  [unwired: 1 in, 2 out]
        n393 = Empty String/Path?(string/path=w777) -> (empty?=w776:bool)
        n394 = case shown="False" w776 {
          tunnel: w779 -> [w804 _]
          tunnel: w778 -> [w803 _]
          tunnel: w777 -> [w795 _]
          frame False {
            # "Valid String"
            n395 = Spreadsheet String To Array(delimiter (Tab)=",", format string="", spreadsheet string=w803, array type (2D Dbl)=i32[] []) -> (array=w798:i32[])
            n396 = property class="MCListbox (strict)"(reference=w804) -> (reference out=w800:refnum<vi>, "ItemNames"=w799:string[][], "RowHdrs[]"=w794:string[])  [unwired: 1 in, 1 out]
            n397 = Index Array(array=w798) -> (element #1=w787:i32, element #2=w786:i32)  [unwired: 2 in]
            n398 = Bundle(w787, w786) -> (w785:cluster{i32, i32})  [unwired: 1 in]
            n399 = Cluster To Array(cluster=w785) -> (array=w790:i32[])
            n400 = Array To Spreadsheet String(delimiter (Tab)=",", array=w790, 3:"" ("format string")) -> (spreadsheet string=w784:string)
            n401 = Replace Array Subset(array=w799, new element=w795, index (row)=w787, index (col)=w786) -> (w797:string[][])
            n402 = Replace Array Subset(array=w794, new element #1=w784, index #1=MCListbox_-_Enum."Initial (KD?)" ("MCListbox Enum"), new element #2="", index #2=MCListbox_-_Enum."Initial Text" ("MCListbox Enum")) -> (w783:string[])
            n403 = property class="MCListbox (strict)"(reference=w800, "ItemNames"=w797, "RowHdrs[]"=w783) -> ()  [unwired: 1 in, 2 out]
            n404 = property on="Extra Event From \"Select Foreign Key\"" class="Bool (strict)"("Val(Sgnl)"=TRUE ("Extended Event From \"Select Foreign Key Value Changed\"")) -> ()  [unwired: 2 in, 2 out]
          }
          frame True {
            # "Empty String"
          }
        }
      }
      event "Database Group": Value Change {
        # "Must assign to same DB.\nBecause did not cater for sign-in across different DB"
        n405 = event-data() -> ()  [unwired: 1 in, 6 out]
        n406 = local read "DB.Config.TableGroupType"() -> (w808:string)
        n407 = local read "DB.Config.TableGroup"() -> (w809:string)
        n408 = call "DB - [Config].[TableGroup].vi"("Table Group Enum"=DB_-_Table_Group_Enum."SELECT [TableGroupId]", "[Description]"="Database Group", "DB Connection"=T5 {"Open"=FALSE, "Close"=FALSE}, "DB.Config.TableGroup"=w809, "DB.Config.TableGroupType"=w808, "connection reference"=w806) -> ("SUMMARY"=w805:errorcluster, "data"=w812:string[])  [unwired: 3 in, 1 out]
        n409 = local read "Application"() -> (w810:string)
        n410 = for {
          tunnel: w812 -> [w816] mode=indexing
          tunnel: w810 -> [w818]
          tunnel: [w815] -> w811 mode=indexing
          n411 = Concatenate Strings(w818, "." ("string"), w816) -> (w815:string)
        }
        n412 = local write "DB"(w805) -> ()
        n413 = property on="Table Name" class="CmbBox (strict)"("Strings[]"=w811) -> ()  [unwired: 2 in, 2 out]
      }
    }
    "Statemachine" <- w68
  }
  n414 = disable-structure shown="Disabled" {
    frame Disabled {
      w820 = "%Y-%m-%d %H:%M:%S"  # SQL Server datetime
      n415 = Get Date/Time In Seconds() -> (seconds since 1Jan1904=w821:timestamp)
      n416 = Format Date/Time String(time format string (%c)=w820, seconds (now)=w821) -> (date/time string=w819:string)  [unwired: 1 in]
      "datetime string" <- w819
      n417 = Concatenate Strings("INSERT INTO " ("string"), "(TStamp)" ("string"), " values " ("string"), "('" ("string"), w819, "')" ("string")) -> ()  [unwired: 1 in, 1 out]
    }
    frame Enabled {
    }
  }
  n418 = call <vilib>:"DB Tools Close Connection.vi"("error in (no error)"=w5, "connection reference"=w6) -> ("error out"=→"Close":errorcluster)  [unwired: 5 in]
